vi "ADC Fetch From Digitizing Process.vi"(6 "stop ref":refnum<vi>, 8 "error in":errorcluster, 10 "Is last multiplexing cycle? (True)":bool=TRUE, 11 "adc session in":T3={"niScope"={"channel cfg"=[], "sessions"=[], "multi cards"=FALSE, "channels"=0, "type"=enum."n/a", "memory [B/chn]"=0, "ext. clock [Hz]"=0.0, "samples count"=0, "use streaming"=FALSE, "proc setup"={"packet size [smpl]"=0, "current timeout [s]"=0.0, "blk2blk timeout [s]"=0.0, "event time"=timestamp(0 s since 1904-01-01), "temp sampl T [s]"=0.0, "data queue"=refnum, "stop notifier"=refnum, "proc ref"=refnum}, "sample width [B]"=0, "ranges [V]"=[], "trigger setup"={"coupling"=1, "level [V]"=0.0, "slope"=0, "mode"=enum."Immediate", "pre-trigger [%]"=0.0}, "fs [Hz]"=0.0, "bitres [bit]"=0, "clock source"=enum."VAL_NO_SOURCE"}, "3458A"={"channels"=[], "sync unit"={"VISA"="", "type"=enum."Picotest U6200A"}, "awg unit"={"type"=enum."Agilent 331xxA to 332xxA", "VISA"="", "enable 10MHz ref"=FALSE, "cmi ckd2"={"VISA"="", "clock source"=enum."Auto", "manual ref clk"=FALSE, "ref clock [Hz]"=0.0, "div mode"=enum."Set divisor directly"}, "cmi sync v3"={"VISA"="", "baud rate [bd/s]"=115200, "source"=enum."Auto", "hv range"=enum."1kV", "fsrc is fixed"=FALSE, "fsrc [Hz]"=10000000.0, "freq integ [s]"=1.0, "freq filter"=5, "trig level"=enum."TTL 5V", "chn1 mode"=enum."Source divider", "chn1 level"=enum."Positive 5V", "chn2 mode"=enum."Source divider", "chn2 level"=enum."Positive 5V", "chn2 div"=1, "chn3 mode"=enum."Chn 1 Active", "chn3 level"=enum."Positive 5V", "chn1 div entry"=enum."Calculate nearest divisor from measured fx", "chn1 dev limit [%]"=1.0, "chn1 check dev"=FALSE}, "trigger"={"source"=enum."Immediate", "slope"=enum."POS", "coupling"=enum."DC", "level [V]"=0.0, "hysteresis [V]"=0.0, "pre-trigger [%]"=0.0}, "HMF2500 cfg"={"Baud Rate"=9600, "Parity"=0, "Data Bits"=8, "Flow Control"=4}}, "sync mode"=enum."MASTER-SLAVE, MASTER clocked by TIMER", "streaming mode"=FALSE, "idn mode"=enum."Auto", "sampling mode"=enum."DCV", "sample memory [B]"=0, "proc setup"={"channel id"=0, "packet size [smpl]"=0, "current timeout [s]"=0.0, "blk2blk timeout [s]"=0.0, "event time"=timestamp(0 s since 1904-01-01), "stop notifier"=refnum, "data queues"=[], "proc refs"=[], "bus semaphore"=refnum}, "sample size [B]"=0, "sample count"=0, "aux data"={"channel id"=0, "valid?"=[], "gain [V]"=[], "timestamp [s]"=[], "Ts [s]"=0.0, "abs timestamp"=timestamp(0 s since 1904-01-01), "t [deg C]"=[], "multiplex timestamp [s]"=-1.0, "only multiplex?"=FALSE, "multiplex smpl offset"=0, "overflow?"=FALSE}, "ranges [V]"=[], "aperture [s]"=0.0, "LEVEL trigger"={"edge"=enum."POS", "level [V]"=0.0, "coupling"=enum."DC"}, "trigger mode"=enum."AUTO", "measure temp.?"=FALSE, "disp mesages"=[], "shared bus?"=FALSE, "disable display?"=FALSE, "aper mode"=enum."Manual", "aper rules"=[], "multiplex"={"cycles"=0, "delay [s]"=0.0, "enabled"=FALSE, "overhead [s]"=1.0, "tot smpls"=0, "sub-rec"=0, "overhead [%]"=0.0, "emulated"=FALSE}, "F8588 lpf"=enum."Off", "F8588 pll"=enum."Off", "F8588 couple"=enum."DC, auto", "fs"={"freq mode"=enum."fs or Ts", "fs [Hz]"=0.0, "fref [Hz]"=0.0, "mul"=0.0, "div"=0.0}, "fs mode"=enum."fs or Ts", "init timestamp"=timestamp(0 s since 1904-01-01), "last report timestamp"=timestamp(0 s since 1904-01-01)}, "dsdll"={"dsdll"={"dsdll path"=path "", "dsdll handle"=[], "output devices"=[], "capture devices"=[]}, "channels"=0, "device id"=0, "channel idns"=[], "proc setup"={"packet size [smpl]"=0, "current timeout [s]"=0.0, "blk2blk timeout [s]"=0.0, "event time"=timestamp(0 s since 1904-01-01), "data queue"=refnum, "stop notifier"=refnum, "proc ref"=refnum}, "samples count"=0, "fs [Hz]"=0.0}, "type"=enum."niScope", "channel idn str"=[], "aux instr idn str"=[], "modified?"=FALSE, "simadc"={"channels"=[], "range [V]"=0.0, "Ts step [s]"=0.0, "time [s]"=0.0, "fs [Hz]"=0.0, "count"=0, "smpl offset"=0, "set count"=0, "bit res"=0}, "force rst?"=FALSE, "exit mode"=enum."Immediate reset", "exit dly"=0.0, "exit tmr"=timestamp(0 s since 1904-01-01), "busy?"=FALSE, "accessed?"=FALSE, "multiplex"={"Type"=enum."Dummy", "gen com ssn"={"visa"="", "primary"=enum."None", "secondary"=enum."None", "channels"=[]}, "delay before [s]"=0.0, "delay post [s]"=0.0, "sequence"=[], "enabled"=FALSE, "ref timestamp [s]"=0.0, "idn string"="", "dev niScope"="", "niScope idx"=0, "QPMX ssn"={"visa"="", "switch mode"=enum."Switched by TWM", "sequence"=[], "timing delays"=[], "polarity"=enum."Positive", "ss delay (s)"=2.0, "internal timer (s)"=1.0, "Last loaded sequence file"=path "", "startup delay (s)"=2.0}, "VISA mux ssn"={"VISA"="", "paths"=[], "idn command"="", "serial cfg"={"Baud rate"=9600, "Data bits"=8, "Parity"=0, "Stop bits"=10, "Flow control"=0, "End Mode Read"=enum."None", "End Mode Write"=enum."None", "Term character"=0, "Term enable"=FALSE}}}, "keysight dso"={"VISA"="", "channels"=[], "bw limit [Hz]"=0.0, "resolution"=enum."Basic", "trig noise reject"=enum."Normal", "N"=0, "trigger config"={"trigger source"=enum."Immediate", "trigger slope"=enum."Negative", "level [V]"=0.0, "hysteresis [V]"=0.001, "pre-trig [%]"=50}, "fs [Hz]"=0.0, "timeout stop"=timestamp(0 s since 1904-01-01), "waiting for opc"=FALSE, "fetch offset [smpl]"=0, "abs timestamp"=timestamp(0 s since 1904-01-01), "ranges [V]"=[], "decimation"=1.0, "ext ref"=FALSE, "emulate aperture"=FALSE, "model"=enum."DSO91304"}, "cdaq"={"mclk [Hz]"=12800000.0, "ADC task"="", "mclk reference"="", "fs [Hz]"=50000.0, "queue adc cmd"=refnum, "queue adc data"=refnum, "adc proc ref"=refnum, "channels"=[], "last channels"=[], "timeout"=timestamp(0 s since 1904-01-01), "N"=1000, "mclk mode"=enum."Free running", "ext mclk source"=""}, "ignore overload"=FALSE, "ADS127L21"={"VISA"="", "chn list"=[], "record size"=0, "phys. channels"=0, "adc fifo size"=0, "channels"=[], "ext refclk?"=FALSE, "fs [Hz]"=0.0, "ext refclk [Hz]"=0.0, "meas refclk [Hz]"=0.0, "EXTOUT mode"=enum."ADCCLK", "EXTOUT polarity"=enum."NORM", "EXTOUT divisor"=0}} {"ADS127L21"."channels"."Channel" min=1 max=8 step=1; "ADS127L21"."channels"."Range [Vpk]" items=["±1.65V", "±2V"]; "cdaq"."last channels"."Channel id" min=0 step=1; "cdaq"."channels"."Channel id" min=0 step=1; "keysight dso"."decimation" min=1.0; "keysight dso"."bw limit [Hz]" format="%#_6p"; "keysight dso"."channels"."Offset [V]" format="%#_6p"; "keysight dso"."channels"."Range [Vpk]" min=0.0 format="%#_6p"; "keysight dso"."channels"."Channel" min=1; "multiplex"."VISA mux ssn"."serial cfg"."Flow control" items=["None", "XON/XOFF", "CTS/RTS", "XON/XOFF + CTS/RTS", "DTR/DSR", "XON/XOFF + DTR/DSR"]; "multiplex"."VISA mux ssn"."serial cfg"."Stop bits" items=["1 bit"=10, "1.5 bits"=15, "2 bits"=20]; "multiplex"."VISA mux ssn"."serial cfg"."Parity" items=["None", "Odd", "Even", "Mark", "Space"]; "multiplex"."VISA mux ssn"."serial cfg"."Data bits" items=["5 bits"=5, "6 bits"=6, "7 bits"=7, "8 bits"=8]; "multiplex"."VISA mux ssn"."serial cfg"."Baud rate" items=["150 Bd"=150, "300 Bd"=300, "600 Bd"=600, "1200 Bd"=1200, "2400 Bd"=2400, "4800 Bd"=4800, "9600 Bd"=9600, "19.2 kBd"=19200, "38.4 kBd"=38400, "57.6 kBd"=57600, "115.2 kBd"=115200]; "multiplex"."QPMX ssn"."startup delay (s)" min=0.0 step=1.0; "multiplex"."QPMX ssn"."internal timer (s)" min=0.0 step=1.0; "multiplex"."QPMX ssn"."ss delay (s)" min=0.0 step=1.0; "multiplex"."QPMX ssn"."timing delays" min=1 max=255 step=1; "3458A"."awg unit"."HMF2500 cfg"."Flow Control" items=["None", "XON/XOFF", "RTS/CTS", "XON/XOFF & RTS/CTS", "DTR/DSR", "XON/XOFF & DTR/DSR"]; "3458A"."awg unit"."HMF2500 cfg"."Data Bits" items=["7"=7, "8"=8]; "3458A"."awg unit"."HMF2500 cfg"."Parity" items=["None", "Odd", "Even", "Mark", "Space"]; "3458A"."awg unit"."HMF2500 cfg"."Baud Rate" items=["300"=300, "600"=600, "1200"=1200, "2400"=2400, "4800"=4800, "9600"=9600, "19200"=19200]; "3458A"."awg unit"."cmi sync v3"."chn2 div" min=1 max=100000000 step=1; "3458A"."awg unit"."cmi sync v3"."fsrc [Hz]" format="%_8p"; "3458A"."channels"."Range [Vpk]" min=0.0; "niScope"."trigger setup"."pre-trigger [%]" format="%.2f"; "niScope"."trigger setup"."level [V]" format="%.2f"; "niScope"."trigger setup"."coupling" items=["AC"=0, "DC"=1, "HF Reject"=3, "LF Reject"=4, "AC Plus HF Reject"=1001]; "niScope"."channel cfg"."Range [Vpk]" min=0.0; "niScope"."channel cfg"."Channel" min=0}) -> (0 "error out":errorcluster, 1 "aux data":T1, 2 "data packet":T2, 3 "adc session out":T3={"niScope"={"channel cfg"=[], "sessions"=[], "multi cards"=FALSE, "channels"=0, "type"=enum."n/a", "memory [B/chn]"=0, "ext. clock [Hz]"=0.0, "samples count"=0, "use streaming"=FALSE, "proc setup"={"packet size [smpl]"=0, "current timeout [s]"=0.0, "blk2blk timeout [s]"=0.0, "event time"=timestamp(0 s since 1904-01-01), "temp sampl T [s]"=0.0, "data queue"=refnum, "stop notifier"=refnum, "proc ref"=refnum}, "sample width [B]"=0, "ranges [V]"=[], "trigger setup"={"coupling"=1, "level [V]"=0.0, "slope"=0, "mode"=enum."Immediate", "pre-trigger [%]"=0.0}, "fs [Hz]"=0.0, "bitres [bit]"=0, "clock source"=enum."VAL_NO_SOURCE"}, "3458A"={"channels"=[], "sync unit"={"VISA"="", "type"=enum."Picotest U6200A"}, "awg unit"={"type"=enum."Agilent 331xxA to 332xxA", "VISA"="", "enable 10MHz ref"=FALSE, "cmi ckd2"={"VISA"="", "clock source"=enum."Auto", "manual ref clk"=FALSE, "ref clock [Hz]"=0.0, "div mode"=enum."Set divisor directly"}, "cmi sync v3"={"VISA"="", "baud rate [bd/s]"=115200, "source"=enum."Auto", "hv range"=enum."1kV", "fsrc is fixed"=FALSE, "fsrc [Hz]"=10000000.0, "freq integ [s]"=1.0, "freq filter"=5, "trig level"=enum."TTL 5V", "chn1 mode"=enum."Source divider", "chn1 level"=enum."Positive 5V", "chn2 mode"=enum."Source divider", "chn2 level"=enum."Positive 5V", "chn2 div"=1, "chn3 mode"=enum."Chn 1 Active", "chn3 level"=enum."Positive 5V", "chn1 div entry"=enum."Calculate nearest divisor from measured fx", "chn1 dev limit [%]"=1.0, "chn1 check dev"=FALSE}, "trigger"={"source"=enum."Immediate", "slope"=enum."POS", "coupling"=enum."DC", "level [V]"=0.0, "hysteresis [V]"=0.0, "pre-trigger [%]"=0.0}, "HMF2500 cfg"={"Baud Rate"=9600, "Parity"=0, "Data Bits"=8, "Flow Control"=4}}, "sync mode"=enum."MASTER-SLAVE, MASTER clocked by TIMER", "streaming mode"=FALSE, "idn mode"=enum."Auto", "sampling mode"=enum."DCV", "sample memory [B]"=0, "proc setup"={"channel id"=0, "packet size [smpl]"=0, "current timeout [s]"=0.0, "blk2blk timeout [s]"=0.0, "event time"=timestamp(0 s since 1904-01-01), "stop notifier"=refnum, "data queues"=[], "proc refs"=[], "bus semaphore"=refnum}, "sample size [B]"=0, "sample count"=0, "aux data"={"channel id"=0, "valid?"=[], "gain [V]"=[], "timestamp [s]"=[], "Ts [s]"=0.0, "abs timestamp"=timestamp(0 s since 1904-01-01), "t [deg C]"=[], "multiplex timestamp [s]"=-1.0, "only multiplex?"=FALSE, "multiplex smpl offset"=0, "overflow?"=FALSE}, "ranges [V]"=[], "aperture [s]"=0.0, "LEVEL trigger"={"edge"=enum."POS", "level [V]"=0.0, "coupling"=enum."DC"}, "trigger mode"=enum."AUTO", "measure temp.?"=FALSE, "disp mesages"=[], "shared bus?"=FALSE, "disable display?"=FALSE, "aper mode"=enum."Manual", "aper rules"=[], "multiplex"={"cycles"=0, "delay [s]"=0.0, "enabled"=FALSE, "overhead [s]"=1.0, "tot smpls"=0, "sub-rec"=0, "overhead [%]"=0.0, "emulated"=FALSE}, "F8588 lpf"=enum."Off", "F8588 pll"=enum."Off", "F8588 couple"=enum."DC, auto", "fs"={"freq mode"=enum."fs or Ts", "fs [Hz]"=0.0, "fref [Hz]"=0.0, "mul"=0.0, "div"=0.0}, "fs mode"=enum."fs or Ts", "init timestamp"=timestamp(0 s since 1904-01-01), "last report timestamp"=timestamp(0 s since 1904-01-01)}, "dsdll"={"dsdll"={"dsdll path"=path "", "dsdll handle"=[], "output devices"=[], "capture devices"=[]}, "channels"=0, "device id"=0, "channel idns"=[], "proc setup"={"packet size [smpl]"=0, "current timeout [s]"=0.0, "blk2blk timeout [s]"=0.0, "event time"=timestamp(0 s since 1904-01-01), "data queue"=refnum, "stop notifier"=refnum, "proc ref"=refnum}, "samples count"=0, "fs [Hz]"=0.0}, "type"=enum."niScope", "channel idn str"=[], "aux instr idn str"=[], "modified?"=FALSE, "simadc"={"channels"=[], "range [V]"=0.0, "Ts step [s]"=0.0, "time [s]"=0.0, "fs [Hz]"=0.0, "count"=0, "smpl offset"=0, "set count"=0, "bit res"=0}, "force rst?"=FALSE, "exit mode"=enum."Immediate reset", "exit dly"=0.0, "exit tmr"=timestamp(0 s since 1904-01-01), "busy?"=FALSE, "accessed?"=FALSE, "multiplex"={"Type"=enum."Dummy", "gen com ssn"={"visa"="", "primary"=enum."None", "secondary"=enum."None", "channels"=[]}, "delay before [s]"=0.0, "delay post [s]"=0.0, "sequence"=[], "enabled"=FALSE, "ref timestamp [s]"=0.0, "idn string"="", "dev niScope"="", "niScope idx"=0, "QPMX ssn"={"visa"="", "switch mode"=enum."Switched by TWM", "sequence"=[], "timing delays"=[], "polarity"=enum."Positive", "ss delay (s)"=2.0, "internal timer (s)"=1.0, "Last loaded sequence file"=path "", "startup delay (s)"=2.0}, "VISA mux ssn"={"VISA"="", "paths"=[], "idn command"="", "serial cfg"={"Baud rate"=9600, "Data bits"=8, "Parity"=0, "Stop bits"=10, "Flow control"=0, "End Mode Read"=enum."None", "End Mode Write"=enum."None", "Term character"=0, "Term enable"=FALSE}}}, "keysight dso"={"VISA"="", "channels"=[], "bw limit [Hz]"=0.0, "resolution"=enum."Basic", "trig noise reject"=enum."Normal", "N"=0, "trigger config"={"trigger source"=enum."Immediate", "trigger slope"=enum."Negative", "level [V]"=0.0, "hysteresis [V]"=0.001, "pre-trig [%]"=50}, "fs [Hz]"=0.0, "timeout stop"=timestamp(0 s since 1904-01-01), "waiting for opc"=FALSE, "fetch offset [smpl]"=0, "abs timestamp"=timestamp(0 s since 1904-01-01), "ranges [V]"=[], "decimation"=1.0, "ext ref"=FALSE, "emulate aperture"=FALSE, "model"=enum."DSO91304"}, "cdaq"={"mclk [Hz]"=12800000.0, "ADC task"="", "mclk reference"="", "fs [Hz]"=50000.0, "queue adc cmd"=refnum, "queue adc data"=refnum, "adc proc ref"=refnum, "channels"=[], "last channels"=[], "timeout"=timestamp(0 s since 1904-01-01), "N"=1000, "mclk mode"=enum."Free running", "ext mclk source"=""}, "ignore overload"=FALSE, "ADS127L21"={"VISA"="", "chn list"=[], "record size"=0, "phys. channels"=0, "adc fifo size"=0, "channels"=[], "ext refclk?"=FALSE, "fs [Hz]"=0.0, "ext refclk [Hz]"=0.0, "meas refclk [Hz]"=0.0, "EXTOUT mode"=enum."ADCCLK", "EXTOUT polarity"=enum."NORM", "EXTOUT divisor"=0}} {"ADS127L21"."channels"."Channel" min=1 max=8 step=1; "ADS127L21"."channels"."Range [Vpk]" items=["±1.65V", "±2V"]; "cdaq"."last channels"."Channel id" min=0 step=1; "cdaq"."channels"."Channel id" min=0 step=1; "keysight dso"."decimation" min=1.0; "keysight dso"."bw limit [Hz]" format="%#_6p"; "keysight dso"."channels"."Offset [V]" format="%#_6p"; "keysight dso"."channels"."Range [Vpk]" min=0.0 format="%#_6p"; "keysight dso"."channels"."Channel" min=1; "multiplex"."VISA mux ssn"."serial cfg"."Flow control" items=["None", "XON/XOFF", "CTS/RTS", "XON/XOFF + CTS/RTS", "DTR/DSR", "XON/XOFF + DTR/DSR"]; "multiplex"."VISA mux ssn"."serial cfg"."Stop bits" items=["1 bit"=10, "1.5 bits"=15, "2 bits"=20]; "multiplex"."VISA mux ssn"."serial cfg"."Parity" items=["None", "Odd", "Even", "Mark", "Space"]; "multiplex"."VISA mux ssn"."serial cfg"."Data bits" items=["5 bits"=5, "6 bits"=6, "7 bits"=7, "8 bits"=8]; "multiplex"."VISA mux ssn"."serial cfg"."Baud rate" items=["150 Bd"=150, "300 Bd"=300, "600 Bd"=600, "1200 Bd"=1200, "2400 Bd"=2400, "4800 Bd"=4800, "9600 Bd"=9600, "19.2 kBd"=19200, "38.4 kBd"=38400, "57.6 kBd"=57600, "115.2 kBd"=115200]; "multiplex"."QPMX ssn"."startup delay (s)" min=0.0 step=1.0; "multiplex"."QPMX ssn"."internal timer (s)" min=0.0 step=1.0; "multiplex"."QPMX ssn"."ss delay (s)" min=0.0 step=1.0; "multiplex"."QPMX ssn"."timing delays" min=1 max=255 step=1; "3458A"."awg unit"."HMF2500 cfg"."Flow Control" items=["None", "XON/XOFF", "RTS/CTS", "XON/XOFF & RTS/CTS", "DTR/DSR", "XON/XOFF & DTR/DSR"]; "3458A"."awg unit"."HMF2500 cfg"."Data Bits" items=["7"=7, "8"=8]; "3458A"."awg unit"."HMF2500 cfg"."Parity" items=["None", "Odd", "Even", "Mark", "Space"]; "3458A"."awg unit"."HMF2500 cfg"."Baud Rate" items=["300"=300, "600"=600, "1200"=1200, "2400"=2400, "4800"=4800, "9600"=9600, "19200"=19200]; "3458A"."awg unit"."cmi sync v3"."chn2 div" min=1 max=100000000 step=1; "3458A"."awg unit"."cmi sync v3"."fsrc [Hz]" format="%_8p"; "3458A"."channels"."Range [Vpk]" min=0.0; "niScope"."trigger setup"."pre-trigger [%]" format="%.2f"; "niScope"."trigger setup"."level [V]" format="%.2f"; "niScope"."trigger setup"."coupling" items=["AC"=0, "DC"=1, "HF Reject"=3, "LF Reject"=4, "AC Plus HF Reject"=1001]; "niScope"."channel cfg"."Range [Vpk]" min=0.0; "niScope"."channel cfg"."Channel" min=0}, 4 "fetching done?":bool)   [LabVIEW 2020]
doc: "Call this in a loop to fetch sample data comming from running digitizing process(es). It fetches the sample data, merges them from particular channels to one array.\nIf some sample data are available or a status is updated it will be found in 'data packet' variable. Content of the variable is valid only if its flag 'valid?' is true. It contains data either in int32 or int16 format. Everytime some data are returned the 'count' of samples per channels is non-zero and 'offset' indicates relative position of first sample to the start of sampling. When digitizer is sampling (not just returning data) the flag 'sampling' is true. If supported by selected HW it will also return usage of intrument memory buffer and sample data queue. If not supported the value will be NaN. \nSecond output of the VI is 'aux data' which are returned only once per whole fetching sequence. It is valid if its flag 'valid?' is True. The aux. data contains 'gain' and 'offset' scaling factors needed to convert integer sample data to voltage. It will also return vector of measured temperatures and corresponding timestamps of measurement during the sampling if it is supported by the HW. Last parameter is a relative timestamp of first sample for each channel. \nCaller must check and process content of both 'data packet' and 'aux data' every time this VI is called. Fetching must be terminated when the function returnes error or returnes True on 'fetching done?' flag.\nVI modifies session content so do not assign just ADC session in!"
uses:
  ADC Session.ctl
  drivers/niScope/niScope Session.ctl
  drivers/niScope/niScope Virtual Channel Config.ctl
  drivers/niScope/niScope Virtual Channel Mode.ctl
  drivers/niScope/niScope Virtual Channel Input Z.ctl
  drivers/niScope/niScope Virtual Channel Coupling.ctl
  drivers/niScope/niScope Type.ctl
  drivers/niScope/niScope Digitizing Process Options.ctl
  drivers/niScope/niScope Data Packet.ctl
  drivers/niScope/niScope Trigger Setup.ctl
  <instrlib>/niScope/Controls/niScope trigger coupling.ctl
  <instrlib>/niScope/Controls/niScope trigger slope.ctl
  drivers/niScope/niScope Reference Clock.ctl
  drivers/DMM/3458A Digitizer Session.ctl
  drivers/DMM/3458A Virtual Channel Config.ctl
  drivers/Counter/Counter Session.ctl
  drivers/Counter/Counter Type.ctl
  drivers/AWG/AWG Session.ctl
  drivers/AWG/AWG Type.ctl
  drivers/AWG/CMI Clock Divider v2/CMI ckd2 Session.ctl
  drivers/AWG/CMI Clock Divider v2/CMI ckd2 Source Mode.ctl
  drivers/AWG/CMI Clock Divider v2/CMI ckd2 Divisor Mode.ctl
  drivers/AWG/CMI Sync V3/CMI Sync V3 session.ctl
  drivers/AWG/CMI Sync V3/Configure/CMI Sync V3 Reference Clock Source.ctl
  drivers/AWG/CMI Sync V3/Configure/CMI Sync V3 HV input Range.ctl
  drivers/AWG/CMI Sync V3/Configure/CMI Sync V3 Trigger Input Level.ctl
  drivers/AWG/CMI Sync V3/Configure/CMI Sync V3 Channel 1 Mode.ctl
  drivers/AWG/CMI Sync V3/Configure/CMI Sync V3 Channel Output Levels.ctl
  drivers/AWG/CMI Sync V3/Configure/CMI Sync V3 Channel 2 Mode.ctl
  drivers/AWG/CMI Sync V3/Configure/CMI Sync V3 Channel 3 Mode.ctl
  drivers/AWG/CMI Sync V3/Configure/CMI Sync V3 Channel 1 Divisor Entry Mode.ctl
  ADC Trig Config.ctl
  ADC Trig Mode Source.ctl
  ADC Trig Slope.ctl
  ADC Trig Coupling.ctl
  drivers/AWG/RaS HMF2500/HMF2500 Config.ctl
  drivers/DMM/3458A Sync Mode.ctl
  drivers/DMM/3458A Idn Mode.ctl
  drivers/DMM/3458A Digitizing Low Levels/Configure/Sampling Mode.ctl
  drivers/DMM/3458A Digitizing Process Options.ctl
  drivers/DMM/3458A Data Packet.ctl
  drivers/DMM/3458A Aux Record Data.ctl
  drivers/DMM/3458A Digitizing Low Levels/Configure/Level Setup.ctl
  drivers/DMM/3458A Digitizing Low Levels/Configure/First Sample Trigger.ctl
  drivers/DMM/3458A Aperture Selection Mode.ctl
  drivers/DMM/3458A Multiplexing Config.ctl
  drivers/Fluke 8588A/F8588A Low Pass Filter.ctl
  drivers/Fluke 8588A/F8588A Phase Lock.ctl
  drivers/Fluke 8588A/F8588A Coupling.ctl
  drivers/DMM/3458A Sampling Rate.ctl
  drivers/AWG/AWG Clock Setup Mode.ctl
  drivers/DMM/3458A Sample Rate Mode.ctl
  drivers/dsdll/DSDLL Session.ctl
  drivers/dsdll/dsdll/dsdll_instance.ctl
  drivers/dsdll/dsdll/dsdll_device_record.ctl
  drivers/dsdll/DSDLL Process Config.ctl
  drivers/dsdll/DSDLL Data Packet.ctl
  ADC Type.ctl
  drivers/simulated_adc/SimAdc Config.ctl
  drivers/simulated_adc/SimAdc Channel Cfg.ctl
  ADC On Close Action.ctl
  Multiplexer/MPX Session.ctl
  Multiplexer/MPX Type.ctl
  drivers/Multiplexers/Generic COM/GCOMM Session.ctl
  drivers/Multiplexers/Generic COM/GCOMM Signal.ctl
  drivers/Multiplexers/Generic COM/GCOMM Virtual Channel.ctl
  drivers/Multiplexers/Generic COM/GCOMM Logic State.ctl
  drivers/Multiplexers/Generic COM/QPMX Session.ctl
  drivers/Multiplexers/QPMX/QPMX switch mode.ctl
  drivers/Multiplexers/QPMX/QPMX polarity.ctl
  drivers/Multiplexers/Generic VISA commands/GVISA Mux Session.ctl
  drivers/Multiplexers/Generic VISA commands/GVISA Mux Path Entry.ctl
  drivers/Multiplexers/Generic VISA commands/met_serial_setup.ctl
  drivers/Agilent DSO 90000/Virtual Digitizer/KeDSO session.ctl
  drivers/Agilent DSO 90000/Virtual Digitizer/KeDSO Virtual Channel.ctl
  drivers/Agilent DSO 90000/Virtual Digitizer/KeDSO High Resolution Mode.ctl
  drivers/Agilent DSO 90000/Virtual Digitizer/KeDSO Trigger Setup.ctl
  drivers/Agilent DSO 90000/Virtual Digitizer/KeDSO Trigger Source.ctl
  drivers/Agilent DSO 90000/Public/Utility/DSO type.ctl
  drivers/cdaq/cDAQ Session.ctl
  drivers/cdaq/low_level_old/cdaq_anal_adc_command.ctl
  drivers/cdaq/low_level_old/cdaq_anal_adc_data.ctl
  drivers/cdaq/cDAQ Virtual Channel.ctl
  drivers/cdaq/cDAQ Master Clock Mode.ctl
  drivers/CMI_ADS127L21/CMI ADS127L21 - Session.ctl
  drivers/CMI_ADS127L21/CMI ADS127L21 - Record Channel.ctl
  drivers/CMI_ADS127L21/CMI ADS127L21 - Input Range.ctl
  drivers/CMI_ADS127L21/CMI ADS127L21 - Input Mode.ctl
  drivers/CMI_ADS127L21/CMI ADS127L21 - Input Impedance.ctl
  drivers/CMI_ADS127L21/CMI ADS127L21 - EXTOUT Mode.ctl
  drivers/CMI_ADS127L21/CMI ADS127L21 - EXTOUT Polarity.ctl
  ADC Data Packet.ctl
  ADC Aux Data.ctl
  drivers/niScope/niScope Virtual Digitizer.lvlib
  drivers/DMM/3458A Virtual Digitizer.lvlib
  drivers/dsdll/DSDLL Virtual Digitizer.lvlib
  <vilib>/Utility/error.llb/Error Cluster From Error Code.vi
  <vilib>/ErrorRing/Error Ring.xnode
  drivers/Counter/Counter.lvlib
  drivers/AWG/AWG.lvlib
  drivers/DMM/3458A Digitizing Low Levels/3458A Digitizing Low Levels.lvlib
  drivers/dsdll/dsdll/dsdll.lvlib
  drivers/AWG/CMI Sync V3/CMI Sync Unit V3.lvlib
  drivers/Agilent DSO 90000/Agilent 90000 Series.lvlib
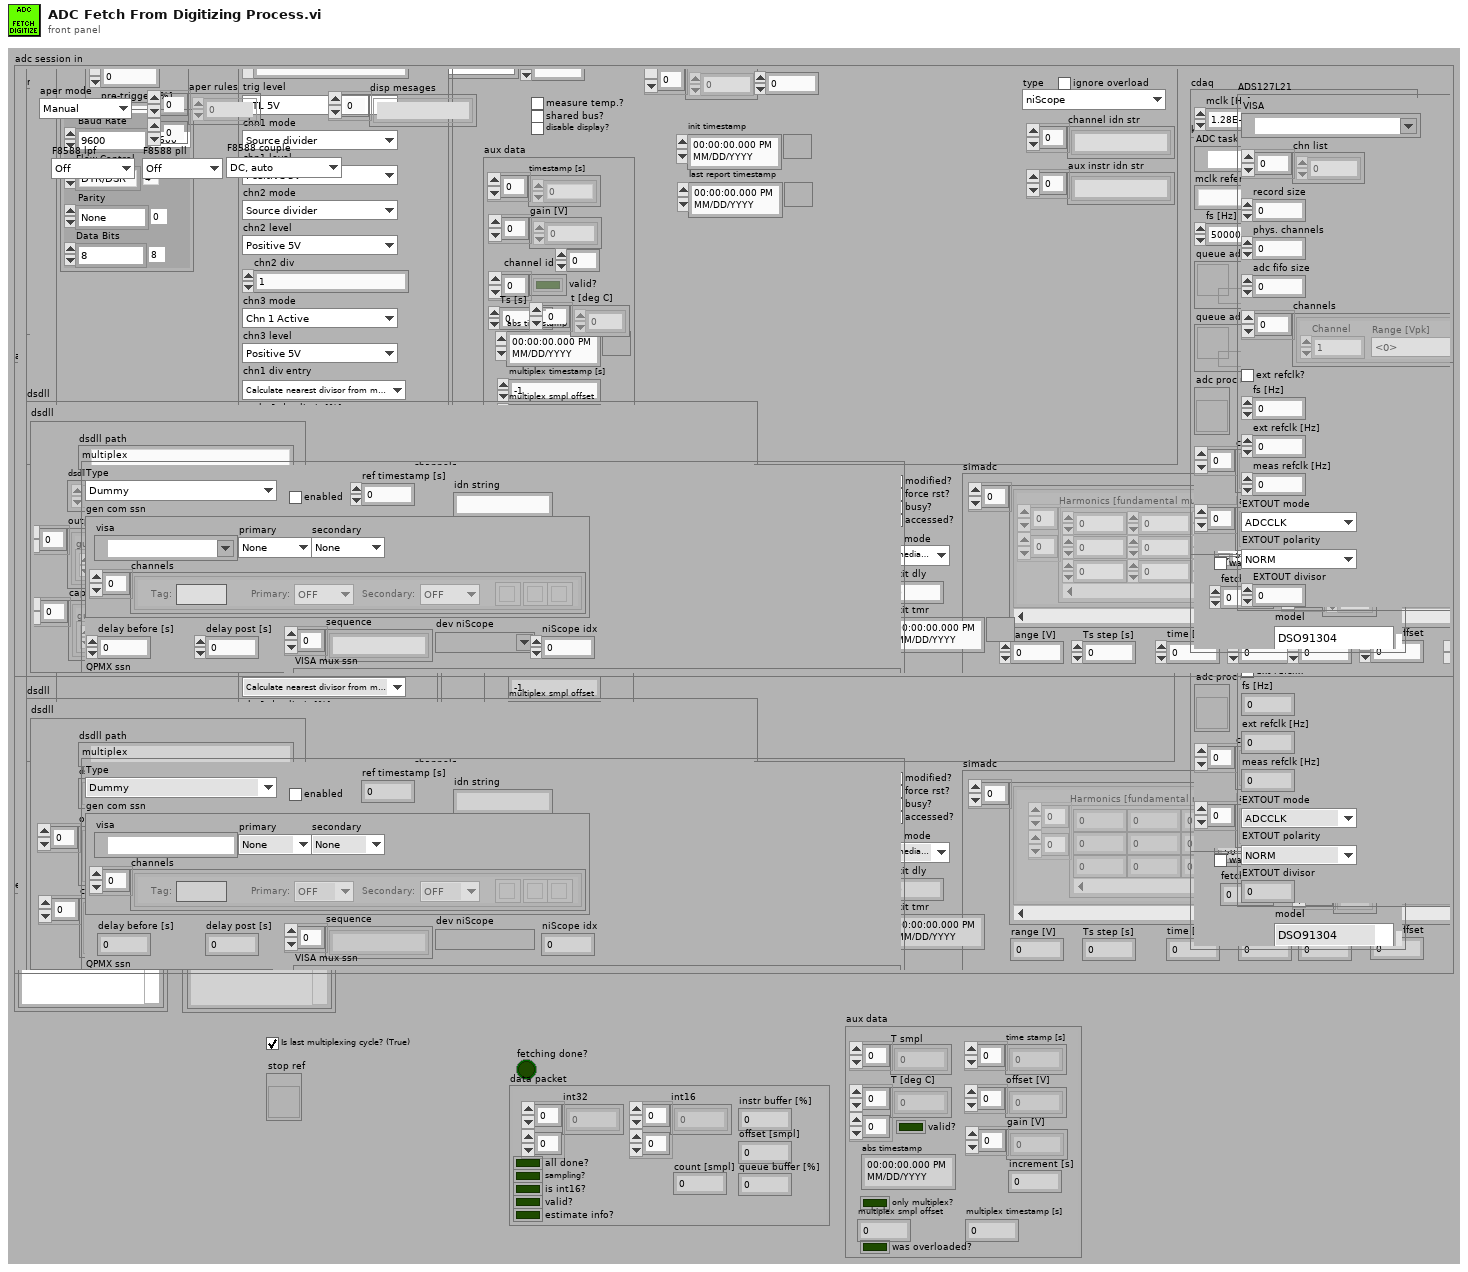
[diagram p1: front panel]
types:
  T1 = typedef "ADC Aux Data.ctl" = cluster{"offset [V]":dbl[], "gain [V]":dbl[], "time stamp [s]":dbl[], "increment [s]":dbl, "T smpl":i64[], "T [deg C]":dbl[][], "valid?":bool, "abs timestamp":timestamp, "only multiplex?":bool, "multiplex smpl offset":i64, "multiplex timestamp [s]":dbl, "was overloaded?":bool}
  T2 = typedef "ADC Data Packet.ctl" = cluster{"int32":i32[][], "int16":i16[][], "offset [smpl]":i64, "count [smpl]":i32, "is int16?":bool, "all done?":bool, "sampling?":bool, "instr buffer [%]":dbl, "queue buffer [%]":dbl, "valid?":bool, "estimate info?":bool}
  T3 = typedef "ADC Session.ctl" = cluster{"niScope":T4, "3458A":T15, "dsdll":T54, "type":T58, "channel idn str":string[], "aux instr idn str":string[], "modified?":bool, "simadc":T59, "force rst?":bool, "exit mode":T61, "exit dly":dbl, "exit tmr":timestamp, "busy?":bool, "accessed?":bool, "multiplex":T62, "keysight dso":T74, "cdaq":T80, "ignore overload":bool, "ADS127L21":T83}
  T4 = typedef "niScope Virtual Digitizer.lvlib/niScope Session.ctl" = cluster{"channel cfg":T5[], "sessions":refnum<k20>[], "multi cards":bool, "channels":i32, "type":T9, "memory [B/chn]":i32, "ext. clock [Hz]":dbl, "samples count":i64, "use streaming":bool, "proc setup":T10, "sample width [B]":i32, "ranges [V]":dbl[], "trigger setup":T11, "fs [Hz]":dbl, "bitres [bit]":i32, "clock source":T14}
  T5 = typedef "niScope Virtual Digitizer.lvlib/niScope Virtual Channel Config.ctl" = cluster{"Address":refnum<k15>, "Channel":i32, "Mode":T6, "Input Z":T7, "Coupling":T8, "Range [Vpk]":dbl, "btn clr":bool, "btn up":bool, "btn down":bool}
  T6 = typedef "niScope Virtual Digitizer.lvlib/niScope Virtual Channel Mode.ctl" = enum16{"Single ended", "Unbal. differential", "Differential"}
  T7 = typedef "niScope Virtual Digitizer.lvlib/niScope Virtual Channel Input Z.ctl" = enum16{"1 MOhm", "50 Ohm"}
  T8 = typedef "niScope Virtual Digitizer.lvlib/niScope Virtual Channel Coupling.ctl" = enum16{"AC", "DC", "GND"}
  T9 = typedef "niScope Virtual Digitizer.lvlib/niScope Type.ctl" = enum16{"n/a", "5922"}
  T10 = typedef "niScope Virtual Digitizer.lvlib/niScope Digitizing Process Options.ctl" = cluster{"packet size [smpl]":i64, "current timeout [s]":dbl, "blk2blk timeout [s]":dbl, "event time":timestamp, "temp sampl T [s]":dbl, "data queue":refnum<queue>, "stop notifier":refnum<notifier>, "proc ref":refnum<vi>}
  T11 = typedef "niScope Virtual Digitizer.lvlib/niScope Trigger Setup.ctl" = cluster{"coupling":T12, "level [V]":dbl, "slope":T13, "mode":enum16{"Immediate", "External", "Level"}, "pre-trigger [%]":dbl}
  T12 = typedef "niScope trigger coupling.ctl" = u16
  T13 = typedef "niScope trigger slope.ctl" = i32
  T14 = typedef "niScope Virtual Digitizer.lvlib/niScope Reference Clock.ctl" = enum16{"VAL_NO_SOURCE", "VAL_CLK_IN", "VAL_PXI_CLOCK", "VAL_EXTERNAL"}
  T15 = typedef "3458A Virtual Digitizer.lvlib/3458A Digitizer Session.ctl" = cluster{"channels":T16[], "sync unit":T17, "awg unit":T19, "sync mode":T38, "streaming mode":bool, "idn mode":T39, "sampling mode":T40, "sample memory [B]":i32, "proc setup":T41, "sample size [B]":i32, "sample count":i32, "aux data":T43, "ranges [V]":dbl[], "aperture [s]":dbl, "LEVEL trigger":T44, "trigger mode":T45, "measure temp.?":bool, "disp mesages":string[], "shared bus?":bool, "disable display?":bool, "aper mode":T46, "aper rules":dbl[][], "multiplex":T47, "F8588 lpf":T48, "F8588 pll":T49, "F8588 couple":T50, "fs":T51, "fs mode":T53, "init timestamp":timestamp, "last report timestamp":timestamp}
  T16 = typedef "3458A Virtual Digitizer.lvlib/3458A Virtual Channel Config.ctl" = cluster{"VISA":refnum<visa-resource-name>, "Range [Vpk]":dbl, "btn clr":bool, "btn up":bool, "btn down":bool, "F8588":bool, "F8588 guard":bool}
  T17 = typedef "Counter.lvlib/Counter Session.ctl" = cluster{"VISA":refnum<visa-resource-name>, "type":T18}
  T18 = typedef "Counter.lvlib/Counter Type.ctl" = enum16{"Picotest U6200A", "dummy"}
  T19 = typedef "AWG.lvlib/AWG Session.ctl" = cluster{"type":T20, "VISA":refnum<visa-resource-name>, "enable 10MHz ref":bool, "cmi ckd2":T21, "cmi sync v3":T24, "trigger":T33, "HMF2500 cfg":T37}
  T20 = typedef "AWG.lvlib/AWG Type.ctl" = enum16{"Agilent 331xxA to 332xxA", "Agilent 335xxA to 336xxA", "Tektronix AFG3101C", "R&S HMF25xx", "CMI Clock Divider v2", "CMI Sync Unit V3", "dummy"}
  T21 = typedef "AWG.lvlib/CMI ckd2 Session.ctl" = cluster{"VISA":refnum<visa-resource-name>, "clock source":T22, "manual ref clk":bool, "ref clock [Hz]":dbl, "div mode":T23}
  T22 = typedef "AWG.lvlib/CMI ckd2 Source Mode.ctl" = enum16{"Auto", "LF clock", "HF clock", "Internal"}
  T23 = typedef "AWG.lvlib/CMI ckd2 Divisor Mode.ctl" = enum16{"Set divisor directly", "Set divisor by frequency"}
  T24 = typedef "AWG.lvlib/CMI Sync Unit V3.lvlib/CMI Sync V3 session.ctl" = cluster{"VISA":refnum<visa-resource-name>, "baud rate [bd/s]":i32, "source":T25, "hv range":T26, "fsrc is fixed":bool, "fsrc [Hz]":dbl, "freq integ [s]":dbl, "freq filter":i32, "trig level":T27, "chn1 mode":T28, "chn1 level":T29, "chn2 mode":T30, "chn2 level":T29, "chn2 div":i32, "chn3 mode":T31, "chn3 level":T29, "chn1 div entry":T32, "chn1 dev limit [%]":dbl, "chn1 check dev":bool}
  T25 = typedef "AWG.lvlib/CMI Sync Unit V3.lvlib/CMI Sync V3 Reference Clock Source.ctl" = enum16{"Auto", "Internal", "Logic", "Sine", "HV"}
  T26 = typedef "AWG.lvlib/CMI Sync Unit V3.lvlib/CMI Sync V3 HV input Range.ctl" = enum16{"10V", "60V", "250V", "1kV"}
  T27 = typedef "AWG.lvlib/CMI Sync Unit V3.lvlib/CMI Sync V3 Trigger Input Level.ctl" = enum16{"LVCMOS 3V3", "TTL 5V"}
  T28 = typedef "AWG.lvlib/CMI Sync Unit V3.lvlib/CMI Sync V3 Channel 1 Mode.ctl" = enum16{"Source divider", "DDS absolute", "DDS ratio", "DDS ratio M/N"}
  T29 = typedef "AWG.lvlib/CMI Sync Unit V3.lvlib/CMI Sync V3 Channel Output Levels.ctl" = enum16{"Positive 3V3", "Negative 3V3", "Positive 5V", "Negative 5V"}
  T30 = typedef "AWG.lvlib/CMI Sync Unit V3.lvlib/CMI Sync V3 Channel 2 Mode.ctl" = enum16{"Source divider", "Chn 1 divide"}
  T31 = typedef "AWG.lvlib/CMI Sync Unit V3.lvlib/CMI Sync V3 Channel 3 Mode.ctl" = enum16{"Chn 1 Active", "Chn 2 Active", "Chn 1 Trigger", "Chn 2 Trigger", "Gate", "PPS", "10MHz"}
  T32 = typedef "AWG.lvlib/CMI Sync Unit V3.lvlib/CMI Sync V3 Channel 1 Divisor Entry Mode.ctl" = enum16{"Set divisor directly", "Calculate nearest divisor from measured fx"}
  T33 = typedef "ADC Trig Config.ctl" = cluster{"source":T34, "slope":T35, "coupling":T36, "level [V]":dbl, "hysteresis [V]":dbl, "pre-trigger [%]":dbl}
  T34 = typedef "ADC Trig Mode Source.ctl" = enum16{"Immediate", "External", "Level"}
  T35 = typedef "ADC Trig Slope.ctl" = enum16{"POS", "NEG"}
  T36 = typedef "ADC Trig Coupling.ctl" = enum16{"DC", "AC"}
  T37 = typedef "AWG.lvlib/HMF2500 Config.ctl" = cluster{"Baud Rate":u32, "Parity":u16, "Data Bits":u16, "Flow Control":u16}
  T38 = typedef "3458A Virtual Digitizer.lvlib/3458A Sync Mode.ctl" = enum16{"MASTER-SLAVE, MASTER clocked by TIMER", "MASTER-SLAVE, MASTER clocked by AWG", "ALL clocked by AWG", "MASTER-SLAVE, ALL clocked by TIMER", "ALL clocked by AWG with DFLL"}
  T39 = typedef "3458A Virtual Digitizer.lvlib/3458A Idn Mode.ctl" = enum16{"Auto", "Sequential (chn A, chn B, ...)", "From calibration string"}
  T40 = typedef "3458A Virtual Digitizer.lvlib/3458A Digitizing Low Levels.lvlib/Sampling Mode.ctl" = enum16{"DCV", "DSDC", "DSAC"}
  T41 = typedef "3458A Virtual Digitizer.lvlib/3458A Digitizing Process Options.ctl" = cluster{"channel id":i32, "packet size [smpl]":i32, "current timeout [s]":dbl, "blk2blk timeout [s]":dbl, "event time":timestamp, "stop notifier":refnum<notifier>, "data queues":refnum<queue>[], "proc refs":refnum<vi>[], "bus semaphore":T42}
  T42 = typedef "Semaphore RefNum" = refnum<k1>
  T43 = typedef "3458A Virtual Digitizer.lvlib/3458A Aux Record Data.ctl" = cluster{"channel id":i32, "valid?":bool[], "gain [V]":dbl[], "timestamp [s]":dbl[], "Ts [s]":dbl, "abs timestamp":timestamp, "t [deg C]":dbl[], "multiplex timestamp [s]":dbl, "only multiplex?":bool, "multiplex smpl offset":i64, "overflow?":bool}
  T44 = typedef "3458A Virtual Digitizer.lvlib/3458A Digitizing Low Levels.lvlib/Level Setup.ctl" = cluster{"edge":enum16{"POS", "NEG"}, "level [V]":dbl, "coupling":enum16{"DC", "AC"}}
  T45 = typedef "3458A Virtual Digitizer.lvlib/3458A Digitizing Low Levels.lvlib/First Sample Trigger.ctl" = enum16{"AUTO", "EXT", "SYN", "SGL", "HOLD", "LEVEL"}
  T46 = typedef "3458A Virtual Digitizer.lvlib/3458A Aperture Selection Mode.ctl" = enum16{"Manual", "Maximum", "Table"}
  T47 = typedef "3458A Virtual Digitizer.lvlib/3458A Multiplexing Config.ctl" = cluster{"cycles":i32, "delay [s]":dbl, "enabled":bool, "overhead [s]":dbl, "tot smpls":i64, "sub-rec":i32, "overhead [%]":dbl, "emulated":bool}
  T48 = typedef "F8588A Low Pass Filter.ctl" = enum16{"Off", "100 kHz", "3 MHz"}
  T49 = typedef "F8588A Phase Lock.ctl" = enum16{"Off", "1 MHz", "10 MHz"}
  T50 = typedef "F8588A Coupling.ctl" = enum16{"AC, 1 MOhm", "AC, 10 MOhm", "DC, 1 MOhm", "DC, 10 MOhm", "DC, auto"}
  T51 = typedef "3458A Virtual Digitizer.lvlib/3458A Sampling Rate.ctl" = cluster{"freq mode":T52, "fs [Hz]":dbl, "fref [Hz]":dbl, "mul":dbl, "div":dbl}
  T52 = typedef "AWG.lvlib/AWG Clock Setup Mode.ctl" = enum16{"fs or Ts", "fs or Ts with fref", "fref/N", "fref*M/N", "fref*Ratio"}
  T53 = typedef "3458A Sample Rate Mode.ctl" = enum16{"fs or Ts", "fs*M/N"}
  T54 = typedef "DSDLL Virtual Digitizer.lvlib/DSDLL Session.ctl" = cluster{"dsdll":T55, "channels":i32, "device id":i32, "channel idns":string[], "proc setup":T57, "samples count":i32, "fs [Hz]":dbl}
  T55 = typedef "dsdll.lvlib/dsdll_instance.ctl" = cluster{"dsdll path":path, "dsdll handle":u8[], "output devices":T56[], "capture devices":T56[]}
  T56 = typedef "dsdll.lvlib/dsdll_device_record.ctl" = cluster{"guid":u8[], "name":string}
  T57 = typedef "DSDLL Virtual Digitizer.lvlib/DSDLL Process Config.ctl" = cluster{"packet size [smpl]":i32, "current timeout [s]":dbl, "blk2blk timeout [s]":dbl, "event time":timestamp, "data queue":refnum<queue>, "stop notifier":refnum<notifier>, "proc ref":refnum<vi>}
  T58 = typedef "ADC Type.ctl" = enum16{"niScope", "3458A", "DirectSound DLL", "Keysight DSO", "cDAQ ADC", "CMI ADS127L21", "dummy"}
  T59 = typedef "SimAdc Config.ctl" = cluster{"channels":T60[], "range [V]":dbl, "Ts step [s]":dbl, "time [s]":dbl, "fs [Hz]":dbl, "count":i64, "smpl offset":i64, "set count":i64, "bit res":i32}
  T60 = typedef "SimAdc Channel Cfg.ctl" = cluster{"harmonics":dbl[][], "btn clear":bool, "noise":dbl, "fundamental [Hz]":dbl}
  T61 = typedef "ADC On Close Action.ctl" = enum16{"Immediate reset", "Delayed reset"}
  T62 = typedef "MPX Session.ctl" = cluster{"Type":T63, "gen com ssn":T64, "delay before [s]":dbl, "delay post [s]":dbl, "sequence":string[], "enabled":bool, "ref timestamp [s]":dbl, "idn string":string, "dev niScope":refnum<k15>, "niScope idx":i32, "QPMX ssn":T68, "VISA mux ssn":T71}
  T63 = typedef "MPX Type.ctl" = enum16{"Dummy", "Generic - COM port", "Generic - niScope PFI", "Generic - VISA commands", "QPMX"}
  T64 = typedef "GCOMM Session.ctl" = cluster{"visa":refnum<visa-resource-name>, "primary":T65, "secondary":T65, "channels":T66[]}
  T65 = typedef "GCOMM Signal.ctl" = enum16{"None", "DTR", "RTS"}
  T66 = typedef "GCOMM Virtual Channel.ctl" = cluster{"Primary:":T67, "Secondary:":T67, "btn clr":bool, "btn up":bool, "btn down":bool, "Tag:":string}
  T67 = typedef "GCOMM Logic State.ctl" = enum16{"OFF", "ON"}
  T68 = typedef "QPMX Session.ctl" = cluster{"visa":refnum<visa-resource-name>, "switch mode":T69, "sequence":bool[][], "timing delays":u32[], "polarity":T70, "ss delay (s)":dbl, "internal timer (s)":dbl, "Last loaded sequence file":path, "startup delay (s)":dbl}
  T69 = typedef "QPMX switch mode.ctl" = enum16{"Switched by TWM", "Switched by external clock", "Switched by internal clock"}
  T70 = typedef "QPMX polarity.ctl" = enum16{"Positive", "Negative"}
  T71 = typedef "GVISA Mux Session.ctl" = cluster{"VISA":refnum<visa-resource-name>, "paths":T72[], "idn command":string, "serial cfg":T73}
  T72 = typedef "GVISA Mux Path Entry.ctl" = cluster{"Tag:":string, "Command:":string, "btn clr":bool, "btn up":bool, "btn down":bool}
  T73 = typedef "met_serial_setup.ctl" = cluster{"Baud rate":i32, "Data bits":i32, "Parity":i32, "Stop bits":i32, "Flow control":i32, "End Mode Read":enum16{"None", "Last Bit", "TermChar"}, "End Mode Write":enum16{"None", "Last Bit", "TermChar"}, "Term character":u8, "Term enable":bool}
  T74 = typedef "KeDSO session.ctl" = cluster{"VISA":refnum<visa-resource-name>, "channels":T75[], "bw limit [Hz]":dbl, "resolution":T76, "trig noise reject":enum16{"Normal", "High Sensitivity"}, "N":i64, "trigger config":T77, "fs [Hz]":dbl, "timeout stop":timestamp, "waiting for opc":bool, "fetch offset [smpl]":i64, "abs timestamp":timestamp, "ranges [V]":dbl[], "decimation":dbl, "ext ref":bool, "emulate aperture":bool, "model":T79}
  T75 = typedef "KeDSO Virtual Channel.ctl" = cluster{"Channel":i32, "Range [Vpk]":dbl, "btn clr":bool, "btn up":bool, "btn down":bool, "Offset [V]":dbl, "Coupling":enum16{"DC", "DC50", "AC", "LFR1"}, "bw limit enab":bool}
  T76 = typedef "KeDSO High Resolution Mode.ctl" = enum16{"Basic", "High-res AUTO", "Min. 9-bits", "Min. 10-bits", "Min. 11-bits", "Min. 12-bits", "Fixed 11-bits", "Fixed 12-bits", "Fixed 13-bits", "Fixed 14-bits", "Fixed 15-bits", "Fixed 16-bits"}
  T77 = typedef "KeDSO Trigger Setup.ctl" = cluster{"trigger source":T78, "trigger slope":enum16{"Negative", "Positive", "Either"}, "level [V]":dbl, "hysteresis [V]":dbl, "pre-trig [%]":i32}
  T78 = typedef "KeDSO Trigger Source.ctl" = enum16{"Immediate", "Level", "AUX"}
  T79 = typedef "Agilent 90000 Series.lvlib/DSO type.ctl" = enum16{"DSO91304", "DSO91204", "DSO90804", "DSO90604", "DSO90404", "DSO90254", "DSA91304", "DSA91204", "DSA90804", "DSA90604", "DSA90404", "DSA90254", "DSO9104", "DSO9254", "DSO9404", "MSO9104", "MSO9254", "MSO9404", "MSO9064", "DSO9064", "DSOX91604", "DSOX92004", "DSOX92504", "DSOX92804", "DSOX93204", "DSO93004", "DSO9024H", "DSO9054H", "DSO9104H", "DSO9204H", "DSOS054A", "DSOS104A", "DSOS204A", "DSOS254A", "DSOS404A", "DSOS604A", "DSOS804A", "MSOS054A", "MSOS104A", "MSOS204A", "MSOS254A", "MSOS404A", "MSOS604A", "MSOS804A", "DSAX96204Q", "DSOX96204Q", "DSAX95004Q", "DSOX95004Q", "DSAX93304Q", "DSOX93304Q", "DSAX92504Q", "DSOX92504Q", "DSAX92004Q", "DSOX92004Q"}
  T80 = typedef "cDAQ Session.ctl" = cluster{"mclk [Hz]":dbl, "ADC task":refnum<k21>, "mclk reference":string, "fs [Hz]":dbl, "queue adc cmd":refnum<queue>, "queue adc data":refnum<queue>, "adc proc ref":refnum<vi>, "channels":T81[], "last channels":T81[], "timeout":timestamp, "N":i32, "mclk mode":T82, "ext mclk source":tag}
  T81 = typedef "cDAQ Virtual Channel.ctl" = cluster{"Device":tag, "Channel id":i32, "btn clr":bool, "btn up":bool, "btn down":bool}
  T82 = typedef "cDAQ Master Clock Mode.ctl" = enum16{"Free running", "Export master clock", "Import master clock"}
  T83 = typedef "CMI ADS127L21 - Session.ctl" = cluster{"VISA":refnum<visa-resource-name>, "chn list":i32[], "record size":i32, "phys. channels":i32, "adc fifo size":i32, "channels":T84[], "ext refclk?":bool, "fs [Hz]":dbl, "ext refclk [Hz]":dbl, "meas refclk [Hz]":dbl, "EXTOUT mode":T88, "EXTOUT polarity":T89, "EXTOUT divisor":i32}
  T84 = typedef "CMI ADS127L21 - Record Channel.ctl" = cluster{"Range [Vpk]":T85, "Channel":i32, "Mode":T86, "Impedance":T87, "btn clr":bool, "btn up":bool, "btn down":bool}
  T85 = typedef "CMI ADS127L21 - Input Range.ctl" = dbl
  T86 = typedef "CMI ADS127L21 - Input Mode.ctl" = enum16{"Normal", "Inverted", "GND"}
  T87 = typedef "CMI ADS127L21 - Input Impedance.ctl" = enum16{"1M", "1k5"}
  T88 = typedef "CMI ADS127L21 - EXTOUT Mode.ctl" = enum16{"ADCCLK", "REFCLK", "SMPLCLK", "FIRST"}
  T89 = typedef "CMI ADS127L21 - EXTOUT Polarity.ctl" = enum16{"NORM", "INV"}
  T90 = typedef "niScope Virtual Digitizer.lvlib/niScope Record Aux Data.ctl" = cluster{"T smpl":i64[], "T [deg C]":dbl[][], "time stamp [s]":dbl[], "offset":dbl[], "gain":dbl[], "increment [s]":dbl, "valid?":bool, "abs timestamp":timestamp}
  T91 = typedef "niScope Virtual Digitizer.lvlib/niScope Data Packet.ctl" = cluster{"int32":i32[][], "card buffer [%]":dbl, "all done?":bool, "offset [smpl]":i64, "sampling?":bool, "queue buffer [%]":dbl, "int16":i16[][], "is int16?":bool, "count [smpl]":i32, "valid?":bool}
  T92 = typedef "3458A Virtual Digitizer.lvlib/3458A Data Packet.ctl" = cluster{"data":i32[][], "offset [smpl]":i32, "count [smpl]":i32, "all done?":bool, "sampling?":bool, "queue buffer [%]":dbl, "valid?":bool, "overflow?":bool, "estimate info?":bool}
  T93 = typedef "KeDSO Record Aux Data.ctl" = cluster{"offsets [V]":dbl[], "gains [V]":dbl[], "timestamps [s]":dbl[], "abs timestamp":timestamp, "Ts [s]":dbl, "valid?":bool}
  T94 = typedef "KeDSO Record Sample Data.ctl" = cluster{"int16 data":i16[][], "offset [smpl]":i64, "count [smpl]":i64, "all done?":bool, "sampling?":bool, "valid?":bool}
  T95 = typedef "CMI ADS127L21 - Fetch Data.ctl" = cluster{"data":i32[][], "data valid?":bool, "sampling?":bool, "done?":bool, "gains":dbl[], "aux valid?":bool, "timestamps [s]":dbl[], "FIFO state [%]":dbl, "offset [smpl]":i32, "count [smpl]":i32}
  T96 = typedef "cDAQ Record Aux Data.ctl" = cluster{"offsets [V]":dbl[], "gains [V]":dbl[], "timestamps [s]":dbl[], "abs timestamp":timestamp, "Ts [s]":dbl, "valid?":bool}
  T97 = typedef "cDAQ Record Sample Data.ctl" = cluster{"int32 data":i32[][], "offset [smpl]":i64, "count [smpl]":i64, "all done?":bool, "sampling?":bool, "valid?":bool}
  T98 = typedef "DSDLL Virtual Digitizer.lvlib/DSDLL Aux Record Data.ctl" = cluster{"time stamp [s]":dbl[], "gain":dbl[], "increment [s]":dbl, "valid?":bool, "abs timestamp":timestamp}
  T99 = typedef "DSDLL Virtual Digitizer.lvlib/DSDLL Data Packet.ctl" = cluster{"int32":i32[][], "card buffer [%]":dbl, "all done?":bool, "offset [smpl]":i32, "sampling?":bool, "queue buffer [%]":dbl, "count [smpl]":i32, "valid?":bool}
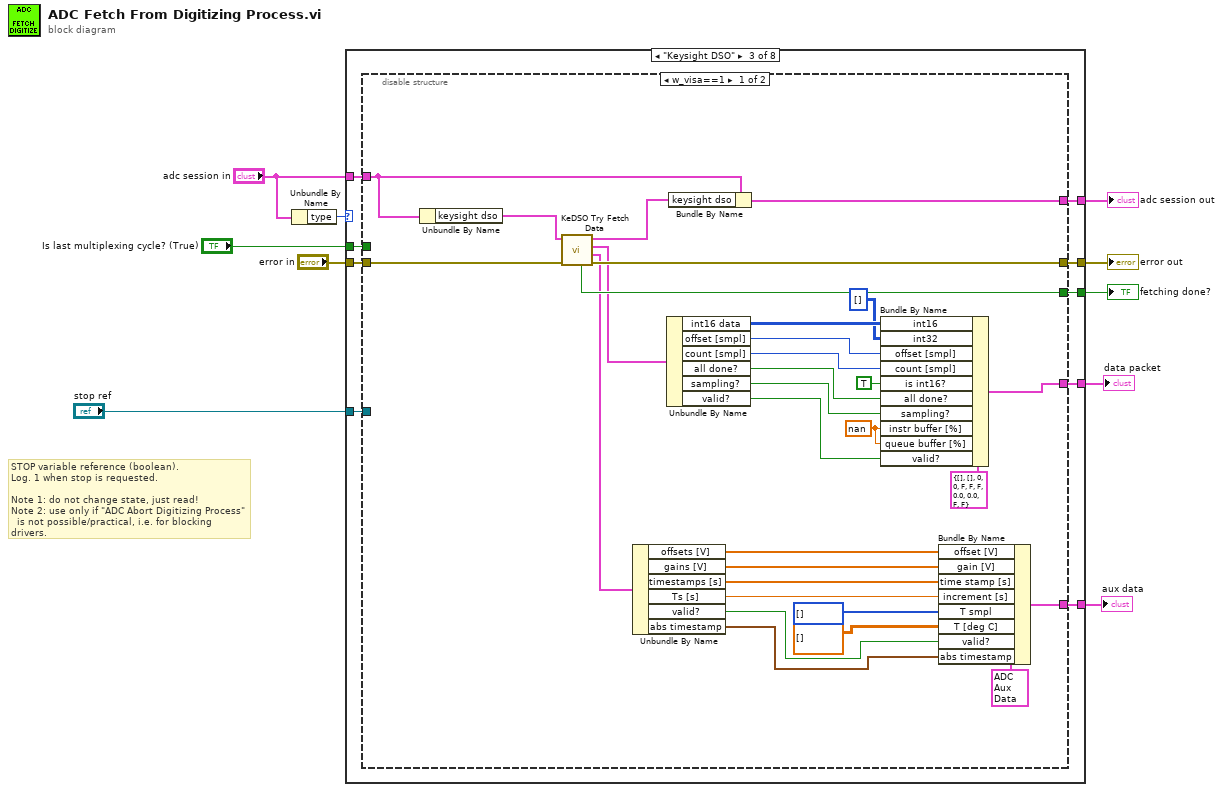
[diagram p0: block diagram]
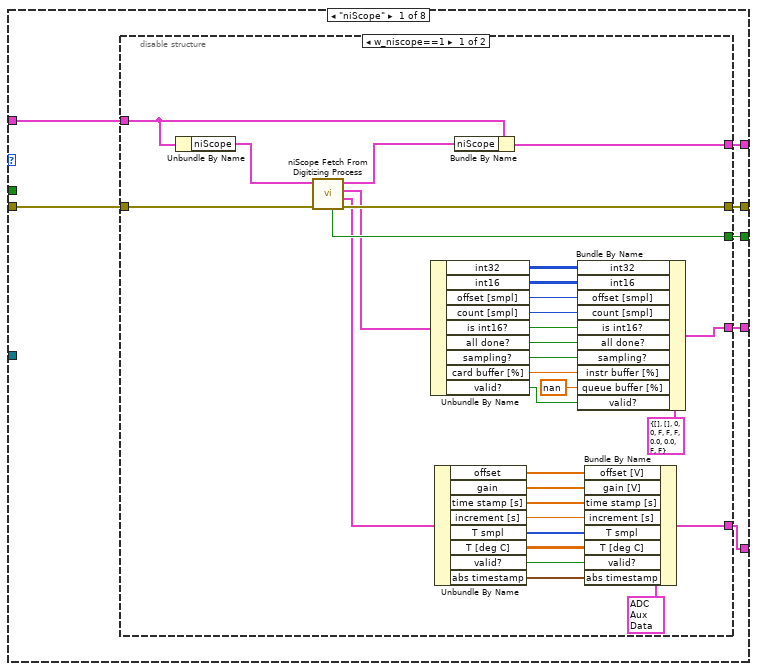
[diagram p2: hidden frame]
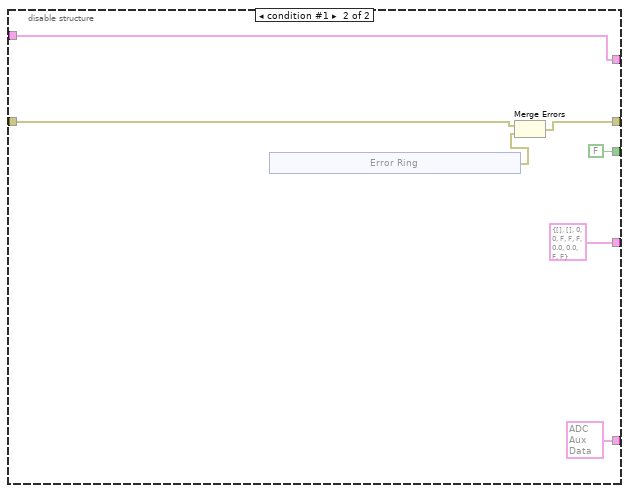
[diagram p3: hidden frame]
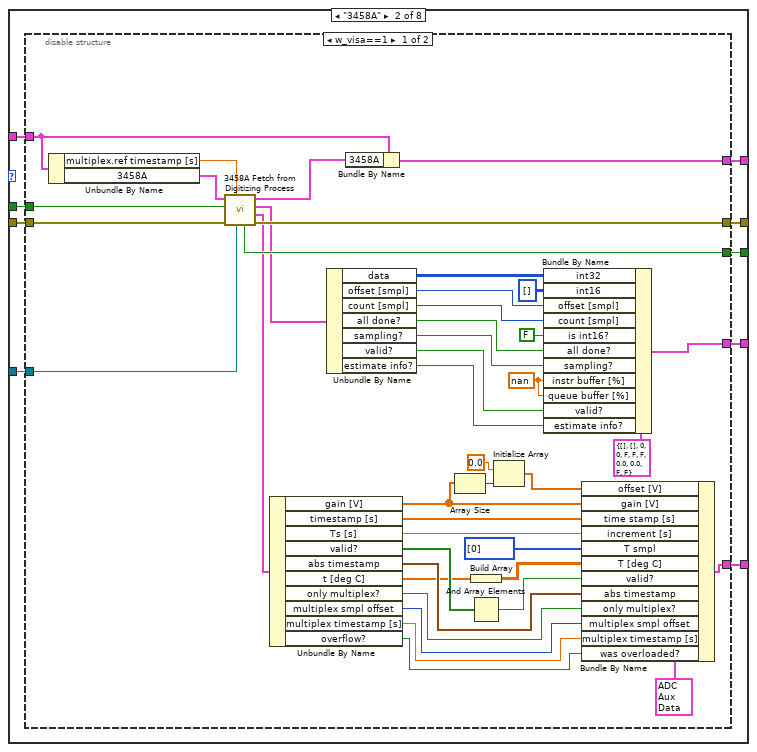
[diagram p4: hidden frame]
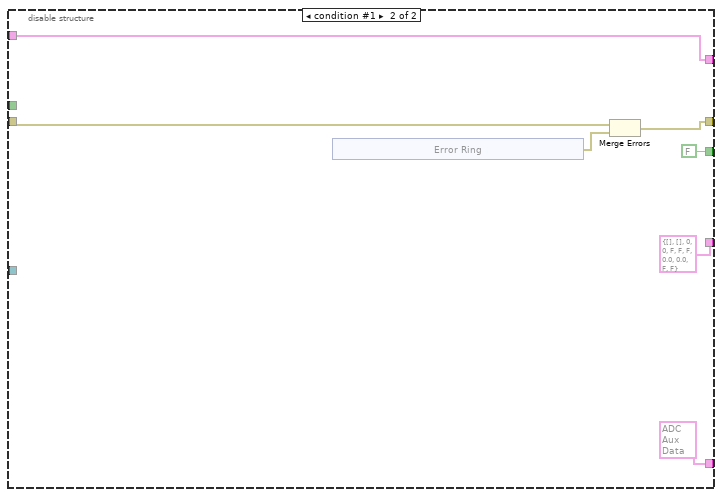
[diagram p5: hidden frame]
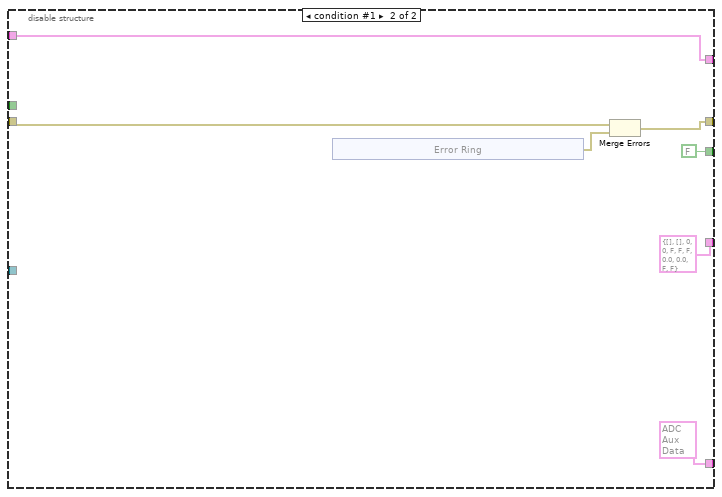
[diagram p6: hidden frame]
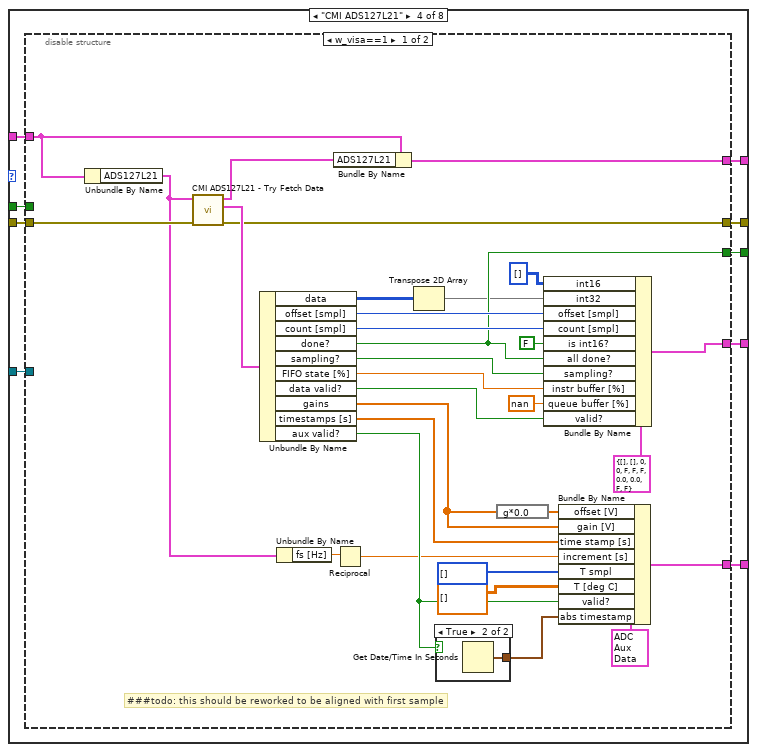
[diagram p7: hidden frame]
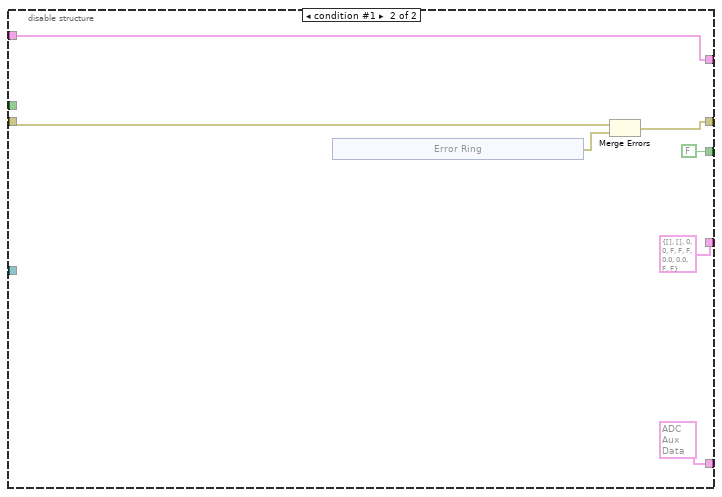
[diagram p9: hidden frame]
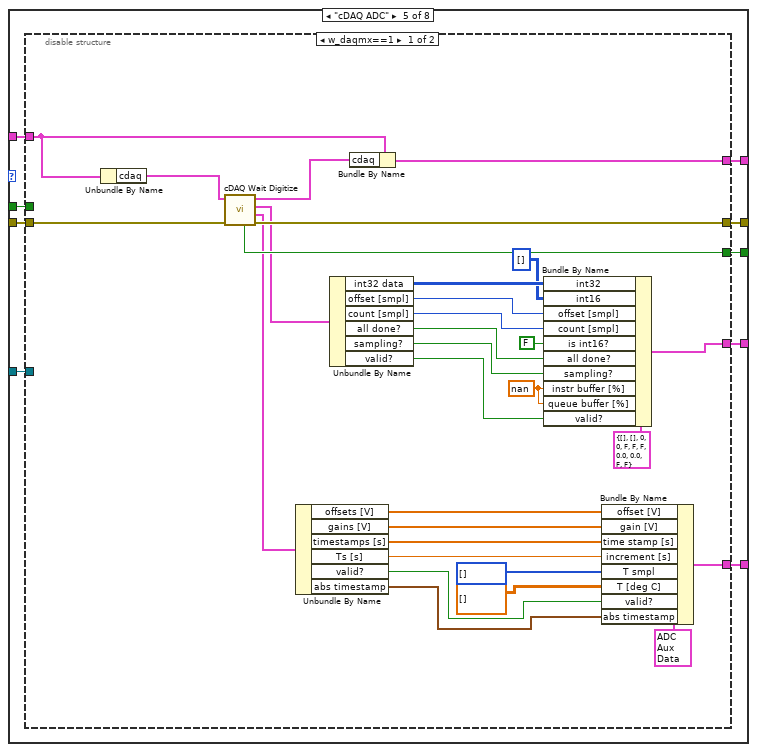
[diagram p10: hidden frame]
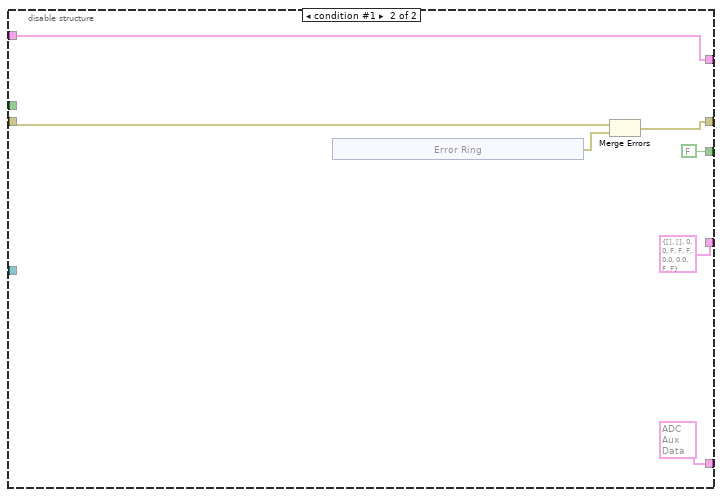
[diagram p11: hidden frame]
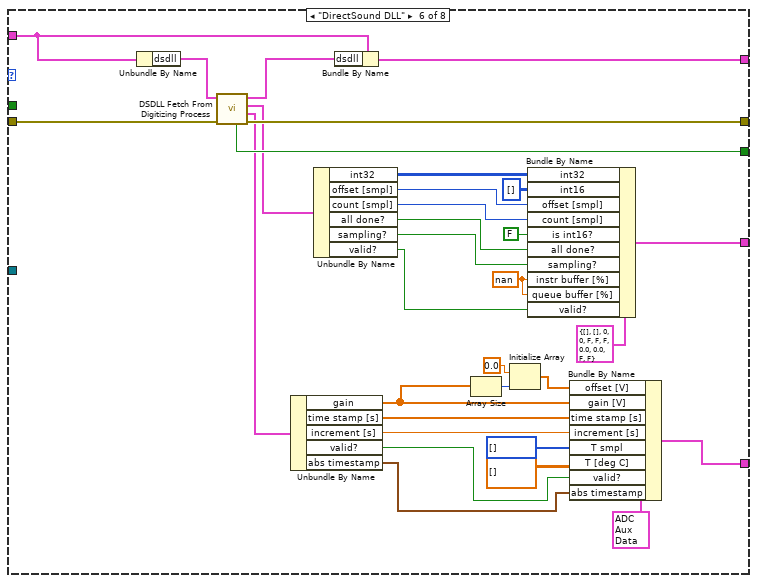
[diagram p12: hidden frame]
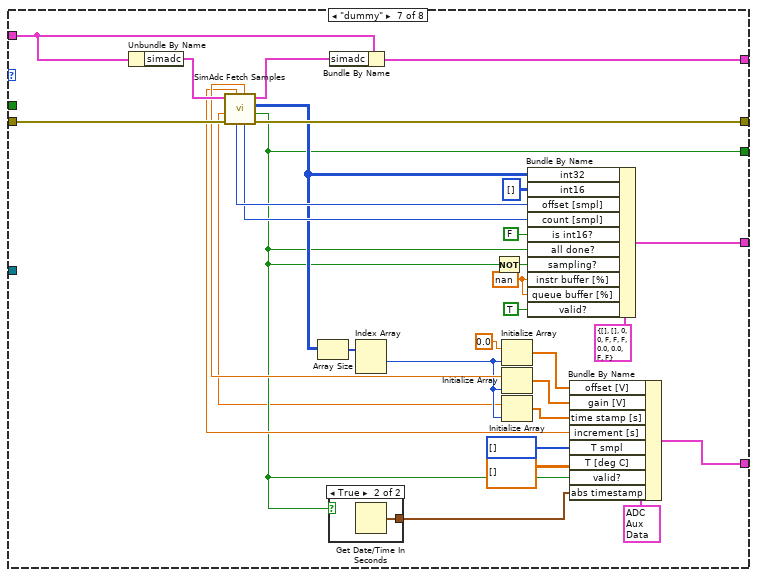
[diagram p13: hidden frame]
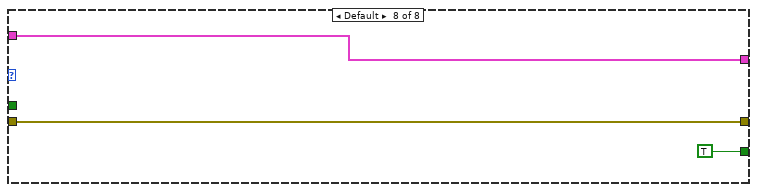
[diagram p15: hidden frame]
diagram:
  # "STOP variable reference (boolean).\nLog. 1 when stop is requested.\n\nNote 1: do not change state, just read!\nNote 2: use only if \"ADC Abort Digitizing Process\"\n  is not possible/practical, i.e. for blocking drivers."
  n1 = Unbundle By Name("adc session in") -> ("type"=w10:T58)
  n2 = case shown="\"Keysight DSO\"" w10 {
    tunnel: "error in" -> [w17 w69 w132 w183 w236 w310 w341 w345]
    tunnel: "adc session in" -> [w16 w68 w131 w182 w235 w308 w339 w344]
    tunnel: [w15 w67 w130 w181 w234 w307 w338 w344] -> w7
    tunnel: [w14 w66 w129 w180 w233 w306 w337 w345] -> w6
    tunnel: [w13 w65 w128 w179 w232 w305 w313 TRUE] -> w5
    tunnel: [w12 w64 w127 w178 w231 w303 w335 _] -> w4
    tunnel: [w11 w63 w126 w177 w230 w292 w330 _] -> w3
    tunnel: "stop ref" -> [_ w62 w125 w176 w229 _ _ _]
    tunnel: "Is last multiplexing cycle? (True)" -> [_ w61 w124 w175 w228 _ _ _]
    frame "niScope" {
      n3 = disable-structure shown="w_niscope==1" {
        disable-tunnel: w17 -> [w48 w54]
        disable-tunnel: w16 -> [w46 w52]
        disable-tunnel: [w44 w52] -> w15
        disable-tunnel: [w43 w53] -> w14
        disable-tunnel: [w42 FALSE ("fetching done?")] -> w13
        disable-tunnel: [w29 T2 {"int32"=[], "int16"=[], "offset [smpl]"=0, "count [smpl]"=0, "is int16?"=FALSE, "all done?"=FALSE, "sampling?"=FALSE, "instr buffer [%]"=0.0, "queue buffer [%]"=0.0, "valid?"=FALSE, "estimate info?"=FALSE} ("data")] -> w12
        disable-tunnel: [w19 T1 {"offset [V]"=[], "gain [V]"=[], "time stamp [s]"=[], "increment [s]"=0.0, "T smpl"=[], "T [deg C]"=[], "valid?"=FALSE, "abs timestamp"=timestamp(0 s since 1904-01-01), "only multiplex?"=FALSE, "multiplex smpl offset"=0, "multiplex timestamp [s]"=0.0, "was overloaded?"=FALSE} ("aux data")] -> w11
        frame condition #0 (active) {
          n4 = Unbundle By Name(w46) -> ("niScope"=w47:T4)
          n5 = call "niScope Fetch From Digitizing Process.vi"("error in"=w48, "niScope in"=w47) -> ("error out"=w43:errorcluster, "auxiliary sampling data"=w28:T90, "data block"=w40:T91, "niScope out"=w45:T4, "fetching done?"=w42:bool)  [unwired: 5 in]
          n6 = Unbundle By Name(w40) -> ("int32"=w39:i32[][], "int16"=w38:i16[][], "offset [smpl]"=w37:i64, "count [smpl]"=w36:i32, "is int16?"=w35:bool, "all done?"=w34:bool, "sampling?"=w33:bool, "card buffer [%]"=w32:dbl, "valid?"=w30:bool)
          n7 = Unbundle By Name(w28) -> ("offset"=w26:dbl[], "gain"=w25:dbl[], "time stamp [s]"=w24:dbl[], "increment [s]"=w23:dbl, "T smpl"=w22:i64[], "T [deg C]"=w21:dbl[][], "valid?"=w20:bool, "abs timestamp"=w18:timestamp)
          n8 = Bundle By Name(cluster=w46, "niScope"=w45) -> (w44:T3)
          n9 = Bundle By Name(cluster=T2 {"int32"=[], "int16"=[], "offset [smpl]"=0, "count [smpl]"=0, "is int16?"=FALSE, "all done?"=FALSE, "sampling?"=FALSE, "instr buffer [%]"=0.0, "queue buffer [%]"=0.0, "valid?"=FALSE, "estimate info?"=FALSE} ("data"), "int32"=w39, "int16"=w38, "offset [smpl]"=w37, "count [smpl]"=w36, "is int16?"=w35, "all done?"=w34, "sampling?"=w33, "instr buffer [%]"=w32, "queue buffer [%]"=nan, "valid?"=w30) -> (w29:T2)
          n10 = Bundle By Name(cluster=T1 {"offset [V]"=[], "gain [V]"=[], "time stamp [s]"=[], "increment [s]"=0.0, "T smpl"=[], "T [deg C]"=[], "valid?"=FALSE, "abs timestamp"=timestamp(0 s since 1904-01-01), "only multiplex?"=FALSE, "multiplex smpl offset"=0, "multiplex timestamp [s]"=0.0, "was overloaded?"=FALSE} ("aux data"), "offset [V]"=w26, "gain [V]"=w25, "time stamp [s]"=w24, "increment [s]"=w23, "T smpl"=w22, "T [deg C]"=w21, "valid?"=w20, "abs timestamp"=w18) -> (w19:T1)
        }
        frame condition #1 {
          n11 = xnode "Error Ring"() -> ("error out"=w55:errorcluster)
          n12 = Merge Errors(w54, w55) -> (w53:errorcluster)
        }
      }
    }
    frame "3458A" {
      n13 = disable-structure shown="w_visa==1" {
        disable-tunnel: w69 -> [w111 w117]
        disable-tunnel: w68 -> [w109 w112]
        disable-tunnel: [w108 w112] -> w67
        disable-tunnel: [w107 w116] -> w66
        disable-tunnel: [w105 FALSE ("fetching done?")] -> w65
        disable-tunnel: [w103 T2 {"int32"=[], "int16"=[], "offset [smpl]"=0, "count [smpl]"=0, "is int16?"=FALSE, "all done?"=FALSE, "sampling?"=FALSE, "instr buffer [%]"=0.0, "queue buffer [%]"=0.0, "valid?"=FALSE, "estimate info?"=FALSE} ("data")] -> w64
        disable-tunnel: [w90 T1 {"offset [V]"=[], "gain [V]"=[], "time stamp [s]"=[], "increment [s]"=0.0, "T smpl"=[], "T [deg C]"=[], "valid?"=FALSE, "abs timestamp"=timestamp(0 s since 1904-01-01), "only multiplex?"=FALSE, "multiplex smpl offset"=0, "multiplex timestamp [s]"=0.0, "was overloaded?"=FALSE} ("aux data")] -> w63
        disable-tunnel: w62 -> [w77 _]
        disable-tunnel: w61 -> [w76 _]
        frame condition #0 (active) {
          w94 = nan ("instr buffer [%]")
          n14 = Unbundle By Name(w109) -> ("multiplex.ref timestamp [s]"=w75:dbl, "3458A"=w106:T15)
          n15 = call "3458A Fetch from Digitizing Process.vi"("stop ref"=w77, "record start timestamp for time multiplex [s]"=w75, "error in"=w111, "Is last multiplexing cycle? (True)"=w76, "session in"=w106) -> ("error out"=w107:errorcluster, "aux data"=w92:T43, "data packet"=w102:T92, "session out"=w110:T15, "fetching done?"=w105:bool)  [unwired: 2 in]
          n16 = Unbundle By Name(w92) -> ("gain [V]"=w84:dbl[], "timestamp [s]"=w89:dbl[], "Ts [s]"=w88:dbl, "valid?"=w86:bool[], "abs timestamp"=w80:timestamp, "t [deg C]"=w79:dbl[], "only multiplex?"=w74:bool, "multiplex smpl offset"=w73:i64, "multiplex timestamp [s]"=w72:dbl, "overflow?"=w71:bool)
          n17 = Unbundle By Name(w102) -> ("data"=w99:i32[][], "offset [smpl]"=w100:i32, "count [smpl]"=w95:i32, "all done?"=w97:bool, "sampling?"=w96:bool, "valid?"=w93:bool, "estimate info?"=w70:bool)
          n18 = Bundle By Name(cluster=w109, "3458A"=w110) -> (w108:T3)
          n19 = Array Size(array=w84) -> (size(s)=w83:i32)
          n20 = Build Array(w79) -> (w78:dbl[][])
          n21 = And Array Elements(Boolean array=w86) -> (logical AND=w85:bool)
          n22 = Initialize Array(0.0 ("offset"), w83) -> (w82:dbl[])
          n23 = Bundle By Name(cluster=T2 {"int32"=[], "int16"=[], "offset [smpl]"=0, "count [smpl]"=0, "is int16?"=FALSE, "all done?"=FALSE, "sampling?"=FALSE, "instr buffer [%]"=0.0, "queue buffer [%]"=0.0, "valid?"=FALSE, "estimate info?"=FALSE} ("data"), "int32"=w99, "int16"=i16[][] [], "offset [smpl]"=w100, "count [smpl]"=w95, "is int16?"=FALSE, "all done?"=w97, "sampling?"=w96, "instr buffer [%]"=w94, "queue buffer [%]"=w94, "valid?"=w93, "estimate info?"=w70) -> (w103:T2)
          n24 = Bundle By Name(cluster=T1 {"offset [V]"=[], "gain [V]"=[], "time stamp [s]"=[], "increment [s]"=0.0, "T smpl"=[], "T [deg C]"=[], "valid?"=FALSE, "abs timestamp"=timestamp(0 s since 1904-01-01), "only multiplex?"=FALSE, "multiplex smpl offset"=0, "multiplex timestamp [s]"=0.0, "was overloaded?"=FALSE} ("aux data"), "offset [V]"=w82, "gain [V]"=w84, "time stamp [s]"=w89, "increment [s]"=w88, "T smpl"=i32[] [0], "T [deg C]"=w78, "valid?"=w85, "abs timestamp"=w80, "only multiplex?"=w74, "multiplex smpl offset"=w73, "multiplex timestamp [s]"=w72, "was overloaded?"=w71) -> (w90:T1)
        }
        frame condition #1 {
          n25 = xnode "Error Ring"() -> ("error out"=w118:errorcluster)
          n26 = Merge Errors(w117, w118) -> (w116:errorcluster)
        }
      }
    }
    frame "Keysight DSO" {
      n27 = disable-structure shown="w_visa==1" {
        disable-tunnel: w132 -> [w162 w168]
        disable-tunnel: w131 -> [w160 w163]
        disable-tunnel: [w159 w163] -> w130
        disable-tunnel: [w158 w167] -> w129
        disable-tunnel: [w157 FALSE ("fetching done?")] -> w128
        disable-tunnel: [w155 T2 {"int32"=[], "int16"=[], "offset [smpl]"=0, "count [smpl]"=0, "is int16?"=FALSE, "all done?"=FALSE, "sampling?"=FALSE, "instr buffer [%]"=0.0, "queue buffer [%]"=0.0, "valid?"=FALSE, "estimate info?"=FALSE} ("data")] -> w127
        disable-tunnel: [w144 T1 {"offset [V]"=[], "gain [V]"=[], "time stamp [s]"=[], "increment [s]"=0.0, "T smpl"=[], "T [deg C]"=[], "valid?"=FALSE, "abs timestamp"=timestamp(0 s since 1904-01-01), "only multiplex?"=FALSE, "multiplex smpl offset"=0, "multiplex timestamp [s]"=0.0, "was overloaded?"=FALSE} ("aux data")] -> w126
        disable-tunnel: w125 -> [_ _]
        disable-tunnel: w124 -> [_ _]
        frame condition #0 (active) {
          w148 = nan ("instr buffer [%]")
          n28 = Unbundle By Name(w160) -> ("keysight dso"=w139:T74)
          n29 = call "KeDSO Try Fetch Data.vi"("error in"=w162, "keysight dso"=w139) -> ("error out"=w158:errorcluster, "aux data"=w146:T93, "sample data"=w154:T94, "keysight dso out"=w161:T74, "fetching done?"=w157:bool)  [unwired: 5 in]
          n30 = Unbundle By Name(w146) -> ("offsets [V]"=w136:dbl[], "gains [V]"=w141:dbl[], "timestamps [s]"=w143:dbl[], "Ts [s]"=w142:dbl, "valid?"=w133:bool, "abs timestamp"=w140:timestamp)
          n31 = Unbundle By Name(w154) -> ("int16 data"=w138:i16[][], "offset [smpl]"=w153:i64, "count [smpl]"=w149:i64, "all done?"=w151:bool, "sampling?"=w150:bool, "valid?"=w147:bool)
          n32 = Bundle By Name(cluster=w160, "keysight dso"=w161) -> (w159:T3)
          n33 = Bundle By Name(cluster=T2 {"int32"=[], "int16"=[], "offset [smpl]"=0, "count [smpl]"=0, "is int16?"=FALSE, "all done?"=FALSE, "sampling?"=FALSE, "instr buffer [%]"=0.0, "queue buffer [%]"=0.0, "valid?"=FALSE, "estimate info?"=FALSE} ("data"), "int16"=w138, "int32"=i32[][] [] ("int16"), "offset [smpl]"=w153, "count [smpl]"=w149, "is int16?"=TRUE, "all done?"=w151, "sampling?"=w150, "instr buffer [%]"=w148, "queue buffer [%]"=w148, "valid?"=w147) -> (w155:T2)
          n34 = Bundle By Name(cluster=T1 {"offset [V]"=[], "gain [V]"=[], "time stamp [s]"=[], "increment [s]"=0.0, "T smpl"=[], "T [deg C]"=[], "valid?"=FALSE, "abs timestamp"=timestamp(0 s since 1904-01-01), "only multiplex?"=FALSE, "multiplex smpl offset"=0, "multiplex timestamp [s]"=0.0, "was overloaded?"=FALSE} ("aux data"), "offset [V]"=w136, "gain [V]"=w141, "time stamp [s]"=w143, "increment [s]"=w142, "T smpl"=i32[] [], "T [deg C]"=dbl[][] [], "valid?"=w133, "abs timestamp"=w140) -> (w144:T1)
        }
        frame condition #1 {
          n35 = xnode "Error Ring"() -> ("error out"=w169:errorcluster)
          n36 = Merge Errors(w168, w169) -> (w167:errorcluster)
        }
      }
    }
    frame "CMI ADS127L21" {
      n37 = disable-structure shown="w_visa==1" {
        disable-tunnel: w183 -> [w204 w221]
        disable-tunnel: w182 -> [w214 w216]
        disable-tunnel: [w213 w216] -> w181
        disable-tunnel: [w192 w220] -> w180
        disable-tunnel: [w189 FALSE ("fetching done?")] -> w179
        disable-tunnel: [w211 T2 {"int32"=[], "int16"=[], "offset [smpl]"=0, "count [smpl]"=0, "is int16?"=FALSE, "all done?"=FALSE, "sampling?"=FALSE, "instr buffer [%]"=0.0, "queue buffer [%]"=0.0, "valid?"=FALSE, "estimate info?"=FALSE} ("data")] -> w178
        disable-tunnel: [w207 T1 {"offset [V]"=[], "gain [V]"=[], "time stamp [s]"=[], "increment [s]"=0.0, "T smpl"=[], "T [deg C]"=[], "valid?"=FALSE, "abs timestamp"=timestamp(0 s since 1904-01-01), "only multiplex?"=FALSE, "multiplex smpl offset"=0, "multiplex timestamp [s]"=0.0, "was overloaded?"=FALSE} ("aux data")] -> w177
        disable-tunnel: w176 -> [_ _]
        disable-tunnel: w175 -> [_ _]
        frame condition #0 (active) {
          # "###todo: this should be reworked to be aligned with first sample"
          n38 = Unbundle By Name(w214) -> ("ADS127L21"=w188:T83)
          n39 = call "CMI ADS127L21 - Try Fetch Data.vi"("error in (no error)"=w204, "ADS127L21 session"=w188) -> ("error out"=w192:errorcluster, "data"=w202:T95, "ADS127L21 session out"=w203:T83)  [unwired: 7 in]
          n40 = Unbundle By Name(w202) -> ("data"=w200:i32[][], "offset [smpl]"=w199:i32, "count [smpl]"=w198:i32, "done?"=w189:bool, "sampling?"=w197:bool, "FIFO state [%]"=w196:dbl, "data valid?"=w195:bool, "gains"=w193:dbl[], "timestamps [s]"=w184:dbl[], "aux valid?"=w190:bool)
          n41 = Unbundle By Name(w188) -> ("fs [Hz]"=w187:dbl)
          n42 = Bundle By Name(cluster=w214, "ADS127L21"=w203) -> (w213:T3)
          n43 = Reciprocal(x=w187) -> (1/x=w186:dbl)
          n44 = Transpose 2D Array(2D array=w200) -> (transposed array=w185:i32[][])
          n45 = case shown="True" w190 {
            tunnel: [_ w215] -> w191
            frame False {
            }
            frame True {
              n46 = Get Date/Time In Seconds() -> (seconds since 1Jan1904=w215:timestamp)
            }
          }
          n47 = expression code="g*0.0"(w193) -> (w194:dbl[])
          n48 = Bundle By Name(cluster=T2 {"int32"=[], "int16"=[], "offset [smpl]"=0, "count [smpl]"=0, "is int16?"=FALSE, "all done?"=FALSE, "sampling?"=FALSE, "instr buffer [%]"=0.0, "queue buffer [%]"=0.0, "valid?"=FALSE, "estimate info?"=FALSE} ("data"), "int16"=i16[][] [], "int32"=w185, "offset [smpl]"=w199, "count [smpl]"=w198, "is int16?"=FALSE, "all done?"=w189, "sampling?"=w197, "instr buffer [%]"=w196, "queue buffer [%]"=nan ("instr buffer [%]"), "valid?"=w195) -> (w211:T2)
          n49 = Bundle By Name(cluster=T1 {"offset [V]"=[], "gain [V]"=[], "time stamp [s]"=[], "increment [s]"=0.0, "T smpl"=[], "T [deg C]"=[], "valid?"=FALSE, "abs timestamp"=timestamp(0 s since 1904-01-01), "only multiplex?"=FALSE, "multiplex smpl offset"=0, "multiplex timestamp [s]"=0.0, "was overloaded?"=FALSE} ("aux data"), "offset [V]"=w194, "gain [V]"=w193, "time stamp [s]"=w184, "increment [s]"=w186, "T smpl"=i32[] [], "T [deg C]"=dbl[][] [], "valid?"=w190, "abs timestamp"=w191) -> (w207:T1)
        }
        frame condition #1 {
          n50 = xnode "Error Ring"() -> ("error out"=w222:errorcluster)
          n51 = Merge Errors(w221, w222) -> (w220:errorcluster)
        }
      }
    }
    frame "cDAQ ADC" {
      n52 = disable-structure shown="w_daqmx==1" {
        disable-tunnel: w236 -> [w266 w272]
        disable-tunnel: w235 -> [w264 w267]
        disable-tunnel: [w263 w267] -> w234
        disable-tunnel: [w262 w271] -> w233
        disable-tunnel: [w261 FALSE ("fetching done?")] -> w232
        disable-tunnel: [w259 T2 {"int32"=[], "int16"=[], "offset [smpl]"=0, "count [smpl]"=0, "is int16?"=FALSE, "all done?"=FALSE, "sampling?"=FALSE, "instr buffer [%]"=0.0, "queue buffer [%]"=0.0, "valid?"=FALSE, "estimate info?"=FALSE} ("data")] -> w231
        disable-tunnel: [w248 T1 {"offset [V]"=[], "gain [V]"=[], "time stamp [s]"=[], "increment [s]"=0.0, "T smpl"=[], "T [deg C]"=[], "valid?"=FALSE, "abs timestamp"=timestamp(0 s since 1904-01-01), "only multiplex?"=FALSE, "multiplex smpl offset"=0, "multiplex timestamp [s]"=0.0, "was overloaded?"=FALSE} ("aux data")] -> w230
        disable-tunnel: w229 -> [_ _]
        disable-tunnel: w228 -> [_ _]
        frame condition #0 (active) {
          w252 = nan ("instr buffer [%]")
          n53 = Unbundle By Name(w264) -> ("cdaq"=w237:T80)
          n54 = call "cDAQ Wait Digitize.vi"("error in"=w266, "cdaq session in"=w237) -> ("error out"=w262:errorcluster, "aux data"=w250:T96, "sample data"=w258:T97, "cdaq session out"=w265:T80, "fetching done?"=w261:bool)  [unwired: 5 in]
          n55 = Unbundle By Name(w250) -> ("offsets [V]"=w241:dbl[], "gains [V]"=w245:dbl[], "timestamps [s]"=w247:dbl[], "Ts [s]"=w246:dbl, "valid?"=w238:bool, "abs timestamp"=w244:timestamp)
          n56 = Unbundle By Name(w258) -> ("int32 data"=w243:i32[][], "offset [smpl]"=w257:i64, "count [smpl]"=w253:i64, "all done?"=w255:bool, "sampling?"=w254:bool, "valid?"=w251:bool)
          n57 = Bundle By Name(cluster=w264, "cdaq"=w265) -> (w263:T3)
          n58 = Bundle By Name(cluster=T2 {"int32"=[], "int16"=[], "offset [smpl]"=0, "count [smpl]"=0, "is int16?"=FALSE, "all done?"=FALSE, "sampling?"=FALSE, "instr buffer [%]"=0.0, "queue buffer [%]"=0.0, "valid?"=FALSE, "estimate info?"=FALSE} ("data"), "int32"=w243, "int16"=i16[][] [], "offset [smpl]"=w257, "count [smpl]"=w253, "is int16?"=FALSE, "all done?"=w255, "sampling?"=w254, "instr buffer [%]"=w252, "queue buffer [%]"=w252, "valid?"=w251) -> (w259:T2)
          n59 = Bundle By Name(cluster=T1 {"offset [V]"=[], "gain [V]"=[], "time stamp [s]"=[], "increment [s]"=0.0, "T smpl"=[], "T [deg C]"=[], "valid?"=FALSE, "abs timestamp"=timestamp(0 s since 1904-01-01), "only multiplex?"=FALSE, "multiplex smpl offset"=0, "multiplex timestamp [s]"=0.0, "was overloaded?"=FALSE} ("aux data"), "offset [V]"=w241, "gain [V]"=w245, "time stamp [s]"=w247, "increment [s]"=w246, "T smpl"=i32[] [], "T [deg C]"=dbl[][] [], "valid?"=w238, "abs timestamp"=w244) -> (w248:T1)
        }
        frame condition #1 {
          n60 = xnode "Error Ring"() -> ("error out"=w273:errorcluster)
          n61 = Merge Errors(w272, w273) -> (w271:errorcluster)
        }
      }
    }
    frame "DirectSound DLL" {
      w295 = nan ("instr buffer [%]")
      n62 = Unbundle By Name(w308) -> ("dsdll"=w285:T54)
      n63 = call "DSDLL Fetch From Digitizing Process.vi"("error in"=w310, "dsdll in"=w285) -> ("error out"=w306:errorcluster, "auxiliary sampling data"=w287:T98, "data block"=w286:T99, "dsdll out"=w309:T54, "fetching done?"=w305:bool)  [unwired: 5 in]
      n64 = Unbundle By Name(w287) -> ("gain"=w281:dbl[], "time stamp [s]"=w291:dbl[], "increment [s]"=w290:dbl, "valid?"=w284:bool, "abs timestamp"=w279:timestamp)
      n65 = Unbundle By Name(w286) -> ("int32"=w300:i32[][], "offset [smpl]"=w301:i32, "count [smpl]"=w296:i32, "all done?"=w298:bool, "sampling?"=w297:bool, "valid?"=w294:bool)
      n66 = Bundle By Name(cluster=w308, "dsdll"=w309) -> (w307:T3)
      n67 = Array Size(array=w281) -> (size(s)=w283:i32)
      n68 = Initialize Array(0.0 ("offset"), w283) -> (w280:dbl[])
      n69 = Bundle By Name(cluster=T2 {"int32"=[], "int16"=[], "offset [smpl]"=0, "count [smpl]"=0, "is int16?"=FALSE, "all done?"=FALSE, "sampling?"=FALSE, "instr buffer [%]"=0.0, "queue buffer [%]"=0.0, "valid?"=FALSE, "estimate info?"=FALSE} ("data"), "int32"=w300, "int16"=i16[][] [], "offset [smpl]"=w301, "count [smpl]"=w296, "is int16?"=FALSE, "all done?"=w298, "sampling?"=w297, "instr buffer [%]"=w295, "queue buffer [%]"=w295, "valid?"=w294) -> (w303:T2)
      n70 = Bundle By Name(cluster=T1 {"offset [V]"=[], "gain [V]"=[], "time stamp [s]"=[], "increment [s]"=0.0, "T smpl"=[], "T [deg C]"=[], "valid?"=FALSE, "abs timestamp"=timestamp(0 s since 1904-01-01), "only multiplex?"=FALSE, "multiplex smpl offset"=0, "multiplex timestamp [s]"=0.0, "was overloaded?"=FALSE} ("aux data"), "offset [V]"=w280, "gain [V]"=w281, "time stamp [s]"=w291, "increment [s]"=w290, "T smpl"=i32[] [], "T [deg C]"=dbl[][] [], "valid?"=w284, "abs timestamp"=w279) -> (w292:T1)
    }
    frame "dummy" {
      w332 = nan ("instr buffer [%]")
      n71 = Unbundle By Name(w339) -> ("simadc"=w321:T59)
      n72 = call "SimAdc Fetch Samples.vi"("error in"=w341, "simadc in"=w321) -> ("error out"=w337:errorcluster, "done"=w313:bool, "sample data"=w320:i32[][], "simadc out"=w340:T59, "samples fetched"=w324:i64, "scale factor [V]"=w318:dbl, "smpl offset"=w325:i64, "Ts [s]"=w314:dbl, "time stamp [s]"=w311:dbl)  [unwired: 1 in]
      n73 = Array Size(array=w320) -> (size(s)=w319:i32[])
      n74 = case shown="True" w313 {
        tunnel: [_ w342] -> w312
        frame False {
        }
        frame True {
          n75 = Get Date/Time In Seconds() -> (seconds since 1Jan1904=w342:timestamp)
        }
      }
      n76 = Bundle By Name(cluster=w339, "simadc"=w340) -> (w338:T3)
      n77 = Index Array(array=w319) -> (element #1=w315:i32)  [unwired: 2 in, 1 out]
      n78 = Not(x=w313) -> (.not. x?=w323:bool)
      n79 = Initialize Array(0.0 ("offset"), w315) -> (w326:dbl[])
      n80 = Initialize Array(w318, w315) -> (w317:dbl[])
      n81 = Initialize Array(w311, w315) -> (w316:dbl[])
      n82 = Bundle By Name(cluster=T2 {"int32"=[], "int16"=[], "offset [smpl]"=0, "count [smpl]"=0, "is int16?"=FALSE, "all done?"=FALSE, "sampling?"=FALSE, "instr buffer [%]"=0.0, "queue buffer [%]"=0.0, "valid?"=FALSE, "estimate info?"=FALSE} ("data"), "int32"=w320, "int16"=i16[][] [], "offset [smpl]"=w325, "count [smpl]"=w324, "is int16?"=FALSE, "all done?"=w313, "sampling?"=w323, "instr buffer [%]"=w332, "queue buffer [%]"=w332, "valid?"=TRUE) -> (w335:T2)
      n83 = Bundle By Name(cluster=T1 {"offset [V]"=[], "gain [V]"=[], "time stamp [s]"=[], "increment [s]"=0.0, "T smpl"=[], "T [deg C]"=[], "valid?"=FALSE, "abs timestamp"=timestamp(0 s since 1904-01-01), "only multiplex?"=FALSE, "multiplex smpl offset"=0, "multiplex timestamp [s]"=0.0, "was overloaded?"=FALSE} ("aux data"), "offset [V]"=w326, "gain [V]"=w317, "time stamp [s]"=w316, "increment [s]"=w314, "T smpl"=i32[] [], "T [deg C]"=dbl[][] [], "valid?"=w313, "abs timestamp"=w312) -> (w330:T1)
    }
    frame Default {
    }
  }
  "error out" <- w6
  "adc session out" <- w7
  "fetching done?" <- w5
  "data packet" <- w4
  "aux data" <- w3
